vi "SIAM-SIMStack_v3.vi"(7 "Constants":T4={"galvox-Line0"=14895, "GalvoX-Blanking"=15500.0, "galvox-count/pix"=-2.474, "Camera-StartLine"=-62, "Camera-Endline"=4000, "Wobbel-total"=4264.0, "SM_ticks"=116, "Trigger_ticks"=100, "galvoxAccel"=5.0, "WobbelAccel"=0.02, "zAccel"=0.05, "z-delay-ticks"=700, "SCMOS-LineSpeed [10µs]"=2.4996, "RS height- Pix"=100, "extra-xgalvo"=83.0, "zcommand"=4026531840, "min turn ticks"=100.0} {"zcommand" format="%x" items=["end_no_ticket"=4027514895, "end_ticket"=4027518991, "NoOp"=4026531840, "Read ticks"=4026535936, "Read ticks to var"=4026535938, "Read IP"=4043313152, "Read IP into var"=4043313154, "Set IP from var"=4043309059, "Set IP from var, relative"=4043313155, "branchRel_if_equal"=4043374849, "decrement_branchRel_if_equal"=4043374945, "decrement_branchRel_if_greaterequal"=4043375201, "decrement_branchRel_if_greaterequal_withTicket"=4043379297, "decrement_branchRel_if_smaller"=4043375457, "increment_branchRel_if_smaller"=4043375473, "readVar"=4060090368, "writeVar"=4060086273, "copyVar0_from_var1"=4060086275, "math_addToVariable"=4076863488, "math_addVToVariable"=4076863489, "math_subToVariable"=4076863490, "math_subVToVariable"=4076863491, "math_multToVariable"=4076863492, "math_multvToVariable"=4076863493, "math_divideToVariable"=4076863494, "math_divideVToVariable"=4076863495, "math_modToVariable"=4076863496, "math_modVToVariable"=4076863497, "logic_and"=4093640704, "logic_or"=4093640706, "logic_xor"=4093640708, "bitshift"=4093640712, "I2C-write"=335544337, "I2C-read"=335548433, "Cam-SPI-write"=3254779905, "UART0-VC-Baud-write"=469958673, "UART0-VC-Baud-read"=469962768, "UART0-VC-write"=469762065, "UART0-VC-write-Var"=469762067, "UART0-VC-read-availabe-bytes-to-var"=470355970, "UART0-VC-read-availabe-bytes"=470355984, "UART0-VC-read-skip-bytes"=469831681, "UART0-VC-read"=469766160, "UART0-VC-read-Var"=469766162, "UART1-TSM-Baud-write"=486735889, "UART1-TSM-Baud-read"=486739984, "UART1-TSM-write"=486539281, "UART1-TSM-write-Var"=486539283, "UART1-TSM-read-availabe-bytes-to-var"=487133186, "UART1-TSM-read-availabe-bytes"=487133200, "UART1-TSM-read-skip-bytes"=486604801, "UART1-TSM-read-skip-bytes"=486608897, "UART1-TSM-read"=486543376, "UART1-TSM-read-Var"=486543378, "UART2-Laser-Baud-write"=503513105, "UART2-Baud-read"=503517200, "UART2-write"=503316497, "UART2-write-Var"=503316499, "UART2-read-availabe-bytes-to-var"=503910402, "UART2-read-availabe-bytes"=503910416, "UART2-read-skip-bytes"=503386113, "UART2-read"=503320592, "UART2-read-Var"=503320594, "UART3-Baud-write"=520290321, "UART3-Baud-read"=520294416, "UART3-write"=520093713, "UART3-write-Var"=520093715, "UART3-read-availabe-bytes-to-var"=520687618, "UART3-read-availabe-bytes"=520687632, "UART3-read-skip-bytes"=520163329, "UART3-read"=520097808, "UART3-read-Var"=520097810, "IO-read_bank0"=3489665024, "IO-write_bank0"=3489660929, "IO-read_bank1"=3506442240, "IO-write_bank1"=3506438145, "DA0-0_LED365"=2684354561, "DA0-1_LED385"=2685403137, "DA0-2_LED440"=2686451713, "DA0-3_LED470"=2687500289, "DA0-4_LED510"=2688548865, "DA0-5_LED550"=2689597441, "DA0-6_LED590"=2690646017, "DA0-7_LED640"=2691694593, "DA1-0_LED-R"=2701131777, "DA1-1_LED-G"=2702180353, "DA1-2_LED-B"=2703228929, "DA1-3_LED-AF"=2704277505, "DA1-4"=2705326081, "DA1-5"=2706374657, "DA1-6"=2707423233, "DA1-7"=2708471809, "DA2-Laser0"=2717908993, "DA2-Laser1"=2718957569, "DA2-Laser2"=2720006145, "DA2-Laser3"=2721054721, "DA2-Laser4"=2722103297, "Analog-read_AD0-0"=2818576384, "Analog-read-store_AD0-0"=2818572290, "AF-Register-transfer r/w"=2835349505, "AF-Register-read"=2835353600, "AF-Register-read-to-var"=2835353602, "AF-Transfer-from-var"=2835349507, "IO-delay_bank0"=3489923073, "IO-delay_bank0_fromVar"=3489923075, "read_cam_clock"=3289124864, "store_cam_clock"=3289120770, "read_cam_phase"=3289190400, "store_cam_phase"=3289186306, "store_cam_phase-t"=3289190402, "r_cam1_NHS"=3254980608, "w_cam1_NHS"=3254976513, "r_cam1_NVS"=3255046144, "w_cam1_NVS"=3255042049, "r_cam1_npx"=3255111680, "w_cam1_npx"=3255107585, "r_cam1_npy"=3255177216, "w_cam1_npy"=3255173121, "r_cam1_xhswait"=3255439360, "w_cam1_xhswait"=3255435265, "r_cam1_xvs_wait"=3255504896, "w_cam1_xvs_wait"=3255500801, "r_cam1_framcounter"=3255570432, "r_cam1_line"=3255635968, "r_cam1_xhs-counter"=3255701504, "r_cam2_NHS"=3271757824, "w_cam2_NHS"=3271753729, "r_cam2_NVS"=3271823360, "w_cam2_NVS"=3271819265, "r_cam2_npx"=3271888896, "w_cam2_npx"=3271884801, "r_cam2_npy"=3271954432, "w_cam2_npy"=3271950337, "r_cam2_xvs_wait"=3272282112, "w_cam2_xvs_wait"=3272278017, "r_cam2_framcounter"=3272347648, "r_cam2_line"=3272413184, "r_cam2_xhs-counter"=3272478720, "start TMSI"=102694919, "set_1Galvo"=101712113, "set_x-Galvo"=102760689, "set_y-Galvo"=103809265, "set_z-Fokus"=104857841, "set_1Galvo_position-only"=101711937, "set_x-Galvo_position-only"=102760513, "set_y-Galvo_position-only"=103809089, "set_z-Fokus_position-only"=104857665, "set_x-Galvo_position-only_ticket"=102764609, "set_y-Galvo_position-only_ticket"=103813185, "set_z-Fokus_position-only_ticket"=104861761, "set_1Galvo_relativ-only"=101712001, "set_x-Galvo_relativ-only"=102760577, "set_y-Galvo_relativ-only"=103809153, "set_z-Fokus_relativ-only"=104857729, "set_1Galvo_speed-only"=101711905, "set_x-Galvo_speed-only"=102760481, "set_y-Galvo_speed-only"=103809057, "set_z-Fokus_speed-only"=104857633, "set_1Galvo_acc-only"=101711889, "set_x-Galvo_acc-only"=102760465, "set_y-Galvo_acc-only"=103809041, "set_z-Fokus_acc-only"=104857617, "read_1Galvo_ticket"=101716032, "read_x-Galvo_ticket"=102764608, "read_y-Galvo_ticket"=103813184, "read_z-Focus_ticket"=104861760, "x-Galvo_pos_fromVar"=102760515, "y-Galvo_pos_fromVar"=103809091, "z-Focus_pos_fromVar"=104857667, "Servo0"=67108865, "Servo0-enable"=68091911, "Servo0-disable"=68091919, "Servo1"=68157441, "Servo1-enable"=69140487, "Servo1-disable"=69140495, "Servo2-enable"=70189063, "Servo2"=69206017, "Servo3-enable"=71237639, "Servo3"=70254593, "x-ssi-init"=202309639, "x-ssi-disable"=202309647, "x-ssi-Bits"=201523201, "x-ssi-Read"=201330688, "x-ssi-ReadToVar"=201326594, "x-ssi-ReadToVar-ticket"=201330690, "y-ssi-init"=203358215, "y-ssi-disable"=203358223, "y-ssi-Bits"=202571777, "y-ssi-Read"=202379264, "y-ssi-ReadToVar"=202375170, "y-ssi-ReadToVat-ticket"=202379266]; "SCMOS-LineSpeed [10µs]" format="%#.6f" items=["EdgeFast-285MHz"=0.9175, "EdgeSlow-95MHz"=2.7525, "Panda4.2"=2.7766, "mer2000"=2.4996]; "galvox-count/pix" format="%#_5f"}, 8 "error in (no error)":errorcluster, 11 "User":T5={"z-distance_motorunits"=100, "#planes"=1, "Digital-out"=enum."Laser1", "NoOfPhaseImages"=7} {"#planes" min=1}) -> (0 "error out":errorcluster, 1 "SIAMScript":T6(array[cluster])=[{"Delay 10µs"=50, "command"=4060086273, "P0"=3, "P1"=1, "P2"=0, "P3"=0, "P4"=0, "P5-ticket"=0, "comment"=""}, {"Delay 10µs"=0, "command"=101711937, "P0"=0, "P1"=160563200, "P2"=0, "P3"=0, "P4"=0, "P5-ticket"=0, "comment"=""}, {"Delay 10µs"=0, "command"=102760513, "P0"=0, "P1"=985958318, "P2"=0, "P3"=0, "P4"=0, "P5-ticket"=0, "comment"=""}, {"Delay 10µs"=0, "command"=3289190402, "P0"=0, "P1"=0, "P2"=0, "P3"=0, "P4"=0, "P5-ticket"=0, "comment"=""}, {"Delay 10µs"=1, "command"=4076863488, "P0"=0, "P1"=381040, "P2"=0, "P3"=0, "P4"=0, "P5-ticket"=0, "comment"=""}, {"Delay 10µs"=0, "command"=4076863492, "P0"=0, "P1"=0, "P2"=0, "P3"=0, "P4"=0, "P5-ticket"=0, "comment"=""}, {"Delay 10µs"=0, "command"=4076863497, "P0"=0, "P1"=1, "P2"=0, "P3"=0, "P4"=0, "P5-ticket"=0, "comment"=""}, {"Delay 10µs"=0, "command"=4076863494, "P0"=0, "P1"=0, "P2"=0, "P3"=0, "P4"=0, "P5-ticket"=0, "comment"=""}, {"Delay 10µs"=0, "command"=4076863488, "P0"=0, "P1"=40, "P2"=0, "P3"=0, "P4"=0, "P5-ticket"=0, "comment"=""}, {"Delay 10µs"=0, "command"=4060086273, "P0"=10, "P1"=-65, "P2"=0, "P3"=0, "P4"=0, "P5-ticket"=0, "comment"=""}, {"Delay 10µs"=0, "command"=4076863492, "P0"=10, "P1"=0, "P2"=0, "P3"=0, "P4"=0, "P5-ticket"=0, "comment"=""}, {"Delay 10µs"=264, "command"=102760481, "P0"=0, "P1"=0, "P2"=-1047728, "P3"=0, "P4"=0, "P5-ticket"=0, "comment"=""}, {"Delay 10µs"=0, "command"=4060086273, "P0"=2, "P1"=7, "P2"=0, "P3"=0, "P4"=0, "P5-ticket"=0, "comment"=""}, {"Delay 10µs"=116, "command"=3489660929, "P0"=2097152, "P1"=2097152, "P2"=0, "P3"=0, "P4"=0, "P5-ticket"=0, "comment"=""}, {"Delay 10µs"=0, "command"=3489660929, "P0"=1, "P1"=1, "P2"=0, "P3"=0, "P4"=0, "P5-ticket"=0, "comment"=""}, {"Delay 10µs"=100, "command"=3489660929, "P0"=1, "P1"=0, "P2"=0, "P3"=0, "P4"=0, "P5-ticket"=0, "comment"=""}, {"Delay 10µs"=12638, "command"=3289190402, "P0"=0, "P1"=0, "P2"=0, "P3"=0, "P4"=0, "P5-ticket"=0, "comment"=""}, {"Delay 10µs"=1, "command"=4076863488, "P0"=0, "P1"=381040, "P2"=0, "P3"=0, "P4"=0, "P5-ticket"=0, "comment"=""}, {"Delay 10µs"=0, "command"=4076863492, "P0"=0, "P1"=0, "P2"=0, "P3"=0, "P4"=0, "P5-ticket"=0, "comment"=""}, {"Delay 10µs"=0, "command"=4076863497, "P0"=0, "P1"=1, "P2"=0, "P3"=0, "P4"=0, "P5-ticket"=0, "comment"=""}, {"Delay 10µs"=0, "command"=4076863494, "P0"=0, "P1"=0, "P2"=0, "P3"=0, "P4"=0, "P5-ticket"=0, "comment"=""}, {"Delay 10µs"=0, "command"=4076863488, "P0"=0, "P1"=40, "P2"=0, "P3"=0, "P4"=0, "P5-ticket"=0, "comment"=""}, {"Delay 10µs"=0, "command"=4060086273, "P0"=10, "P1"=-65, "P2"=0, "P3"=0, "P4"=0, "P5-ticket"=0, "comment"=""}, {"Delay 10µs"=0, "command"=4076863492, "P0"=10, "P1"=0, "P2"=0, "P3"=0, "P4"=0, "P5-ticket"=0, "comment"=""}, {"Delay 10µs"=0, "command"=102760465, "P0"=0, "P1"=794884, "P2"=0, "P3"=0, "P4"=0, "P5-ticket"=0, "comment"=""}, {"Delay 10µs"=0, "command"=101711889, "P0"=0, "P1"=42448, "P2"=0, "P3"=0, "P4"=0, "P5-ticket"=0, "comment"=""}, {"Delay 10µs"=132, "command"=102760465, "P0"=0, "P1"=-794884, "P2"=0, "P3"=0, "P4"=0, "P5-ticket"=0, "comment"=""}, {"Delay 10µs"=0, "command"=101711889, "P0"=0, "P1"=-42448, "P2"=0, "P3"=0, "P4"=0, "P5-ticket"=0, "comment"=""}, {"Delay 10µs"=132, "command"=102760465, "P0"=0, "P1"=0, "P2"=0, "P3"=0, "P4"=0, "P5-ticket"=0, "comment"=""}, {"Delay 10µs"=0, "command"=101711889, "P0"=0, "P1"=0, "P2"=0, "P3"=0, "P4"=0, "P5-ticket"=0, "comment"=""}, {"Delay 10µs"=12855, "command"=3489660929, "P0"=2097152, "P1"=0, "P2"=0, "P3"=0, "P4"=0, "P5-ticket"=0, "comment"=""}, {"Delay 10µs"=70, "command"=4043379297, "P0"=-6, "P1"=2, "P2"=1, "P3"=0, "P4"=0, "P5-ticket"=514, "comment"=""}, {"Delay 10µs"=50, "command"=104857729, "P0"=-25600, "P1"=0, "P2"=0, "P3"=0, "P4"=0, "P5-ticket"=0, "comment"=""}, {"Delay 10µs"=0, "command"=4043379297, "P0"=-43, "P1"=3, "P2"=1, "P3"=0, "P4"=0, "P5-ticket"=515, "comment"=""}, {"Delay 10µs"=50, "command"=104857729, "P0"=25600, "P1"=0, "P2"=0, "P3"=0, "P4"=0, "P5-ticket"=0, "comment"=""}, {"Delay 10µs"=50, "command"=102760513, "P0"=0, "P1"=983040000, "P2"=0, "P3"=0, "P4"=0, "P5-ticket"=0, "comment"=""}, {"Delay 10µs"=10, "command"=4027518991, "P0"=0, "P1"=0, "P2"=0, "P3"=0, "P4"=0, "P5-ticket"=112, "comment"=""}] {"command" format="%x" items=["end_no_ticket"=4027514895, "end_ticket"=4027518991, "NoOp"=4026531840, "Read ticks"=4026535936, "Read ticks to var"=4026535938, "Read IP"=4043313152, "Read IP into var"=4043313154, "Set IP from var"=4043309059, "Set IP from var, relative"=4043313155, "branchRel_if_equal"=4043374849, "decrement_branchRel_if_equal"=4043374945, "decrement_branchRel_if_greaterequal"=4043375201, "decrement_branchRel_if_greaterequal_withTicket"=4043379297, "decrement_branchRel_if_smaller"=4043375457, "increment_branchRel_if_smaller"=4043375473, "readVar"=4060090368, "writeVar"=4060086273, "copyVar0_from_var1"=4060086275, "math_addToVariable"=4076863488, "math_addVToVariable"=4076863489, "math_subToVariable"=4076863490, "math_subVToVariable"=4076863491, "math_multToVariable"=4076863492, "math_multvToVariable"=4076863493, "math_divideToVariable"=4076863494, "math_divideVToVariable"=4076863495, "math_modToVariable"=4076863496, "math_modVToVariable"=4076863497, "logic_and"=4093640704, "logic_or"=4093640706, "logic_xor"=4093640708, "bitshift"=4093640712, "I2C-write"=335544337, "I2C-read"=335548433, "Cam-SPI-write"=3254779905, "UART0-VC-Baud-write"=469958673, "UART0-VC-Baud-read"=469962768, "UART0-VC-write"=469762065, "UART0-VC-write-Var"=469762067, "UART0-VC-read-availabe-bytes-to-var"=470355970, "UART0-VC-read-availabe-bytes"=470355984, "UART0-VC-read-skip-bytes"=469831681, "UART0-VC-read"=469766160, "UART0-VC-read-Var"=469766162, "UART1-TSM-Baud-write"=486735889, "UART1-TSM-Baud-read"=486739984, "UART1-TSM-write"=486539281, "UART1-TSM-write-Var"=486539283, "UART1-TSM-read-availabe-bytes-to-var"=487133186, "UART1-TSM-read-availabe-bytes"=487133200, "UART1-TSM-read-skip-bytes"=486604801, "UART1-TSM-read-skip-bytes"=486608897, "UART1-TSM-read"=486543376, "UART1-TSM-read-Var"=486543378, "UART2-Laser-Baud-write"=503513105, "UART2-Baud-read"=503517200, "UART2-write"=503316497, "UART2-write-Var"=503316499, "UART2-read-availabe-bytes-to-var"=503910402, "UART2-read-availabe-bytes"=503910416, "UART2-read-skip-bytes"=503386113, "UART2-read"=503320592, "UART2-read-Var"=503320594, "UART3-Baud-write"=520290321, "UART3-Baud-read"=520294416, "UART3-write"=520093713, "UART3-write-Var"=520093715, "UART3-read-availabe-bytes-to-var"=520687618, "UART3-read-availabe-bytes"=520687632, "UART3-read-skip-bytes"=520163329, "UART3-read"=520097808, "UART3-read-Var"=520097810, "IO-read_bank0"=3489665024, "IO-write_bank0"=3489660929, "IO-read_bank1"=3506442240, "IO-write_bank1"=3506438145, "DA0-0_LED365"=2684354561, "DA0-1_LED385"=2685403137, "DA0-2_LED440"=2686451713, "DA0-3_LED470"=2687500289, "DA0-4_LED510"=2688548865, "DA0-5_LED550"=2689597441, "DA0-6_LED590"=2690646017, "DA0-7_LED640"=2691694593, "DA1-0_LED-R"=2701131777, "DA1-1_LED-G"=2702180353, "DA1-2_LED-B"=2703228929, "DA1-3_LED-AF"=2704277505, "DA1-4"=2705326081, "DA1-5"=2706374657, "DA1-6"=2707423233, "DA1-7"=2708471809, "DA2-Laser0"=2717908993, "DA2-Laser1"=2718957569, "DA2-Laser2"=2720006145, "DA2-Laser3"=2721054721, "DA2-Laser4"=2722103297, "Analog-read_AD0-0"=2818576384, "Analog-read-store_AD0-0"=2818572290, "AF-Register-transfer r/w"=2835349505, "AF-Register-read"=2835353600, "AF-Register-read-to-var"=2835353602, "AF-Transfer-from-var"=2835349507, "IO-delay_bank0"=3489923073, "IO-delay_bank0_fromVar"=3489923075, "read_cam_clock"=3289124864, "store_cam_clock"=3289120770, "read_cam_phase"=3289190400, "store_cam_phase"=3289186306, "store_cam_phase-t"=3289190402, "r_cam1_NHS"=3254980608, "w_cam1_NHS"=3254976513, "r_cam1_NVS"=3255046144, "w_cam1_NVS"=3255042049, "r_cam1_npx"=3255111680, "w_cam1_npx"=3255107585, "r_cam1_npy"=3255177216, "w_cam1_npy"=3255173121, "r_cam1_xhswait"=3255439360, "w_cam1_xhswait"=3255435265, "r_cam1_xvs_wait"=3255504896, "w_cam1_xvs_wait"=3255500801, "r_cam1_framcounter"=3255570432, "r_cam1_line"=3255635968, "r_cam1_xhs-counter"=3255701504, "r_cam2_NHS"=3271757824, "w_cam2_NHS"=3271753729, "r_cam2_NVS"=3271823360, "w_cam2_NVS"=3271819265, "r_cam2_npx"=3271888896, "w_cam2_npx"=3271884801, "r_cam2_npy"=3271954432, "w_cam2_npy"=3271950337, "r_cam2_xvs_wait"=3272282112, "w_cam2_xvs_wait"=3272278017, "r_cam2_framcounter"=3272347648, "r_cam2_line"=3272413184, "r_cam2_xhs-counter"=3272478720, "start TMSI"=102694919, "set_1Galvo"=101712113, "set_x-Galvo"=102760689, "set_y-Galvo"=103809265, "set_z-Fokus"=104857841, "set_1Galvo_position-only"=101711937, "set_x-Galvo_position-only"=102760513, "set_y-Galvo_position-only"=103809089, "set_z-Fokus_position-only"=104857665, "set_x-Galvo_position-only_ticket"=102764609, "set_y-Galvo_position-only_ticket"=103813185, "set_z-Fokus_position-only_ticket"=104861761, "set_1Galvo_relativ-only"=101712001, "set_x-Galvo_relativ-only"=102760577, "set_y-Galvo_relativ-only"=103809153, "set_z-Fokus_relativ-only"=104857729, "set_1Galvo_speed-only"=101711905, "set_x-Galvo_speed-only"=102760481, "set_y-Galvo_speed-only"=103809057, "set_z-Fokus_speed-only"=104857633, "set_1Galvo_acc-only"=101711889, "set_x-Galvo_acc-only"=102760465, "set_y-Galvo_acc-only"=103809041, "set_z-Fokus_acc-only"=104857617, "read_1Galvo_ticket"=101716032, "read_x-Galvo_ticket"=102764608, "read_y-Galvo_ticket"=103813184, "read_z-Focus_ticket"=104861760, "x-Galvo_pos_fromVar"=102760515, "y-Galvo_pos_fromVar"=103809091, "z-Focus_pos_fromVar"=104857667, "Servo0"=67108865, "Servo0-enable"=68091911, "Servo0-disable"=68091919, "Servo1"=68157441, "Servo1-enable"=69140487, "Servo1-disable"=69140495, "Servo2-enable"=70189063, "Servo2"=69206017, "Servo3-enable"=71237639, "Servo3"=70254593, "x-ssi-init"=202309639, "x-ssi-disable"=202309647, "x-ssi-Bits"=201523201, "x-ssi-Read"=201330688, "x-ssi-ReadToVar"=201326594, "x-ssi-ReadToVar-ticket"=201330690, "y-ssi-init"=203358215, "y-ssi-disable"=203358223, "y-ssi-Bits"=202571777, "y-ssi-Read"=202379264, "y-ssi-ReadToVar"=202375170, "y-ssi-ReadToVat-ticket"=202379266]}, 2 "Camera":T2={"Camera-Expos ms"=0.0, "CameraImages"=7, "cam fps min."=0.0})   [LabVIEW 2011]
uses:
  SIAM_command.ctl
panel:
  in  "calulate values for debug":bool
  out "Waveform Graph":dbl[][](graph)
  in  "Aktiv":T1(array[ring])=[enum."GalvoX", enum."Galvo4"]
  out "phase a":dbl=0.04048114735137636
  out "galvo a":dbl=0.7580607172293603
  out "xGalvoMove":dbl=-12844.599514563108
  out "FrameClock":u32=13119
  out "CamTics":u32=12855
  out "x vel":dbl=-0.9991909385113269
  out "~x-move":dbl=12841.530000000002
  out "~xgalvoend":dbl=2202.999999999998
  out "xgalvostart":dbl=15044.53
  out "expected xduration":dbl=71.67016115511393
  out "expected  Wduration":dbl=264.5751311064591
  out "size(s)":i32=37
  out "WobSubShift":dbl=700.0
  out "Half Turn_ticks":u32=132
  # "version ohne phase!\nversion mit galvo1 parallel galvox!: extra-xgalvo\ntodo: exact interger calculation\ntodo: remove last wobber shift from loop\nlost images? increas min turn ticks\nslow z: increse z-delay"
  # "var 2 =linecounter \nvar 3 =framecounter"
  # "tmsi motor units is *512nm, flumias2020 *~5nm"
  # "<-- user inputs --------------------------- constants ---->"
  # "debug disabled if good working"
  # "15173"
  # "naja nicht immer konstante\nalles count und Pixel und 10µs !!!"
  # "wobbler shift(7)=SQRT(7)*pitch"
  # "lineclock read slow=AD99E =711070 =/256=27.77617"
  # "a gerechnet wobbler~3.7, x~98, eher /10\nz~6ms/2µm"
  # "shift full phase"
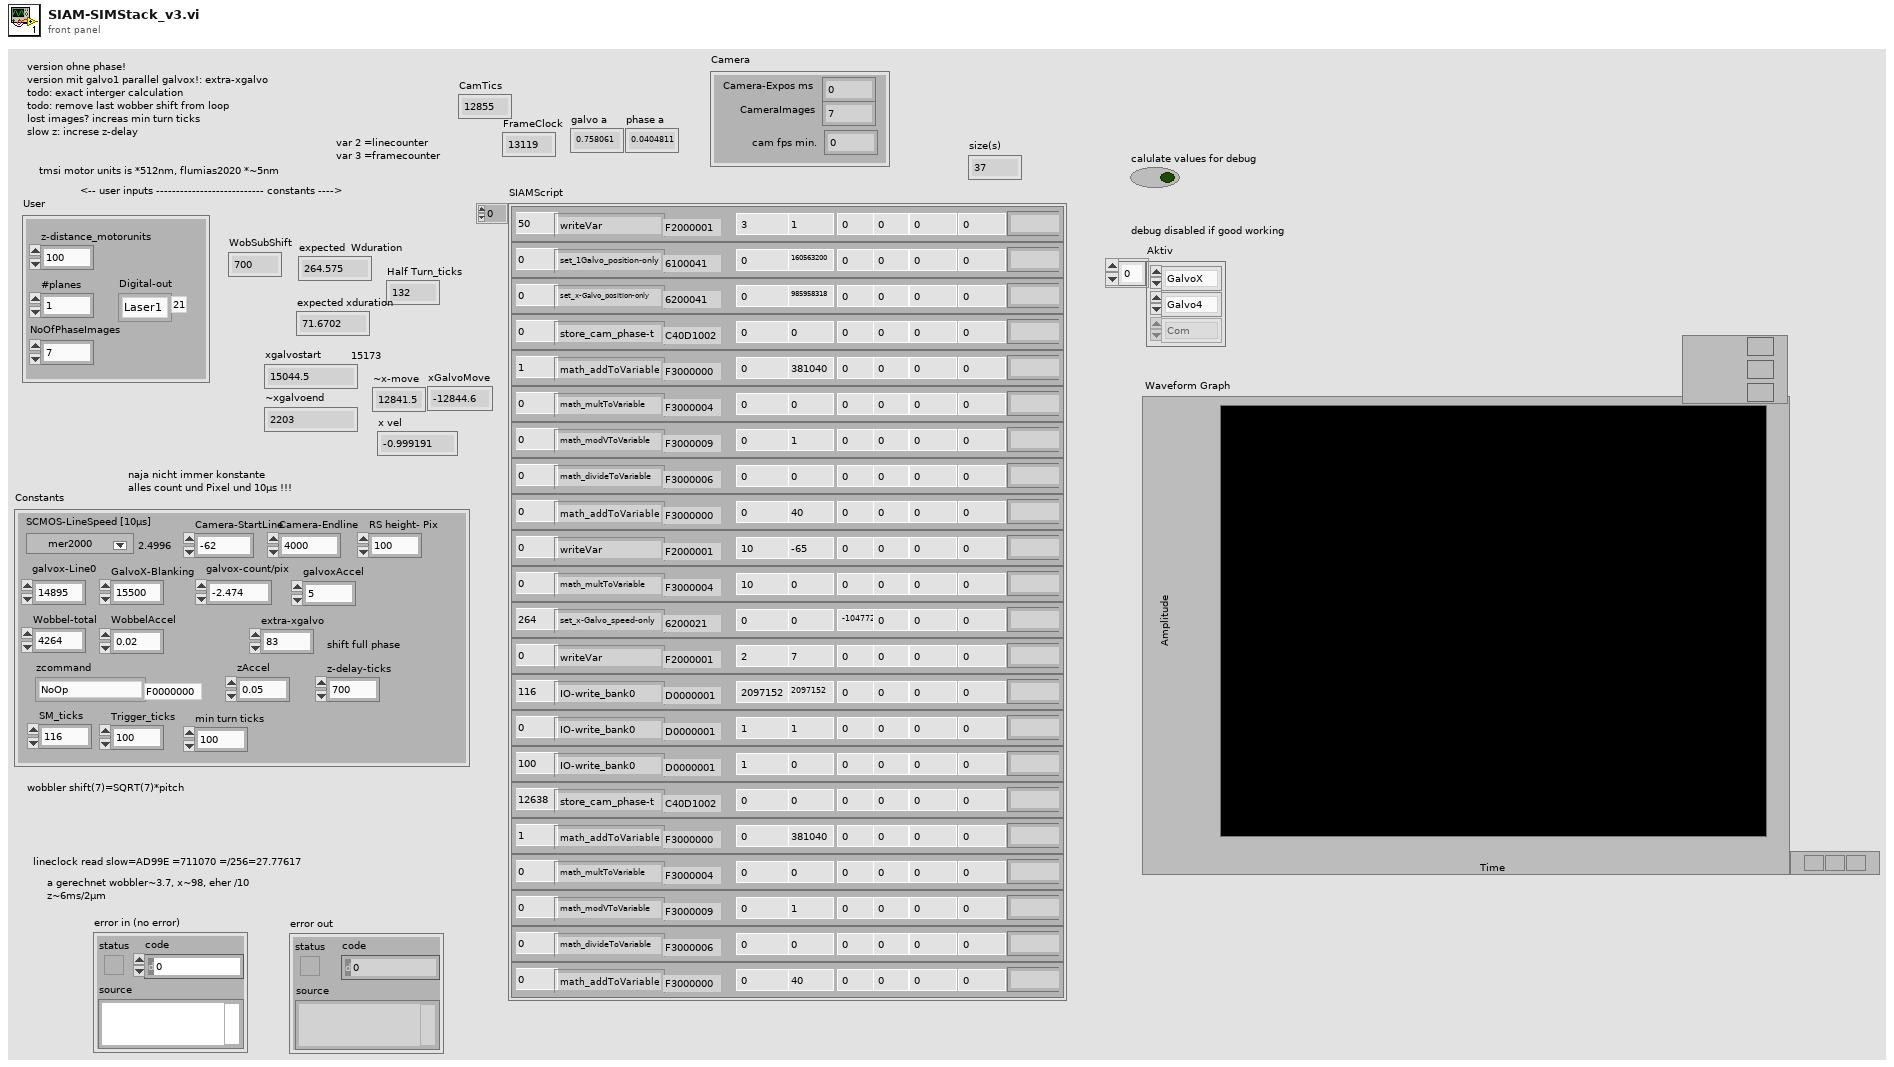
[diagram p1: front panel]
types:
  T1 = enum16{"Com", "AnalogConfig", "AnalogValue", "GalvoX", "GalvoY", "Galvo3", "Galvo4", "Digital", "Free", "Loop", "SMoveTime", "Image1X", "Image1Y", "Image2X", "Image2Y"}[]
  T2 = cluster{"Camera-Expos ms":dbl, "CameraImages":u16, "cam fps min.":dbl}
  T3 = typedef "SIAM_command.ctl" = u32
  T4 = cluster{"galvox-Line0":i16, "GalvoX-Blanking":dbl, "galvox-count/pix":dbl, "Camera-StartLine":i32, "Camera-Endline":u32, "Wobbel-total":dbl, "SM_ticks":u32, "Trigger_ticks":u32, "galvoxAccel":dbl, "WobbelAccel":dbl, "zAccel":dbl, "z-delay-ticks":u32, "SCMOS-LineSpeed [10µs]":dbl, "RS height- Pix":u16, "extra-xgalvo":dbl, "zcommand":T3, "min turn ticks":dbl}
  T5 = cluster{"z-distance_motorunits":i32, "#planes":u16, "Digital-out":enum8{"cam1", "cam1-ready?", "cam2", "cam2-ready?", "tmsx?", "tsmy?", "tsm3?", "lid?", "led1", "led2", "led3", "led4", "led5", "led6", "led7", "led8", "durchR", "durchG", "durchB", "AF", "Laser0", "Laser1", "Laser2", "Laser3", "Laser4", "LaserX", "TrigOut", "SMB1", ""}, "NoOfPhaseImages":u16}
  T6 = cluster{"Delay 10µs":u32, "command":T3, "P0":i32, "P1":i32, "P2":i32, "P3":i32, "P4":i32, "P5-ticket":i32, "comment":string}[]
  T7 = enum8{"Ch0", "Ch1", "x-Galvo", "y-Galvo", "z-Focus"}
  T8 = cluster{"Delay 10µs":u32, "command":T3, "P0":i32, "P1":i32, "P2":i32, "P3":i32, "P4":i32, "P5-ticket":i32, "comment":string}
  T9 = cluster{"Delay 10µs":u32, "command":T3, "P0":i32, "P1":i32, "P2":i32, "P3":i32, "P4":i32, "P5-ticket":i32}[]
  T10 = enum8{"cam1", "cam1-ready?", "cam2", "cam2-ready?", "tmsx?", "tsmy?", "tsm3?", "lid?", "led1", "led2", "led3", "led4", "led5", "led6", "led7", "led8", "durchR", "durchG", "durchB", "AF", "Laser0", "Laser1", "Laser2", "Laser3", "Laser4", "LaserX", "TrigOut", "SMB1", ""}
  T11 = cluster{"Delay 10µs":u32, "command":T3, "P0":i32, "P1":i32, "P2":i32, "P3":i32, "P4":i32, "P5-ticket":i32}
  T12 = typedef "ScanControl_Action.ctl" = enum16{"Abs", "Rel", "Inc", "IncInc", "LoopStart", "LoopEnd", "WaitTriggerRising"}
  T13 = typedef "ScanControl_Channel.ctl" = enum16{"Com", "AnalogConfig", "AnalogValue", "GalvoX", "GalvoY", "Galvo3", "Galvo4", "Digital", "Free", "Loop", "SMoveTime", "Image1X", "Image1Y", "Image2X", "Image2Y"}
  T14 = cluster{"Time [10µs]":dbl, "action":T12, "channel":T13, "value (/s)":dbl}[]
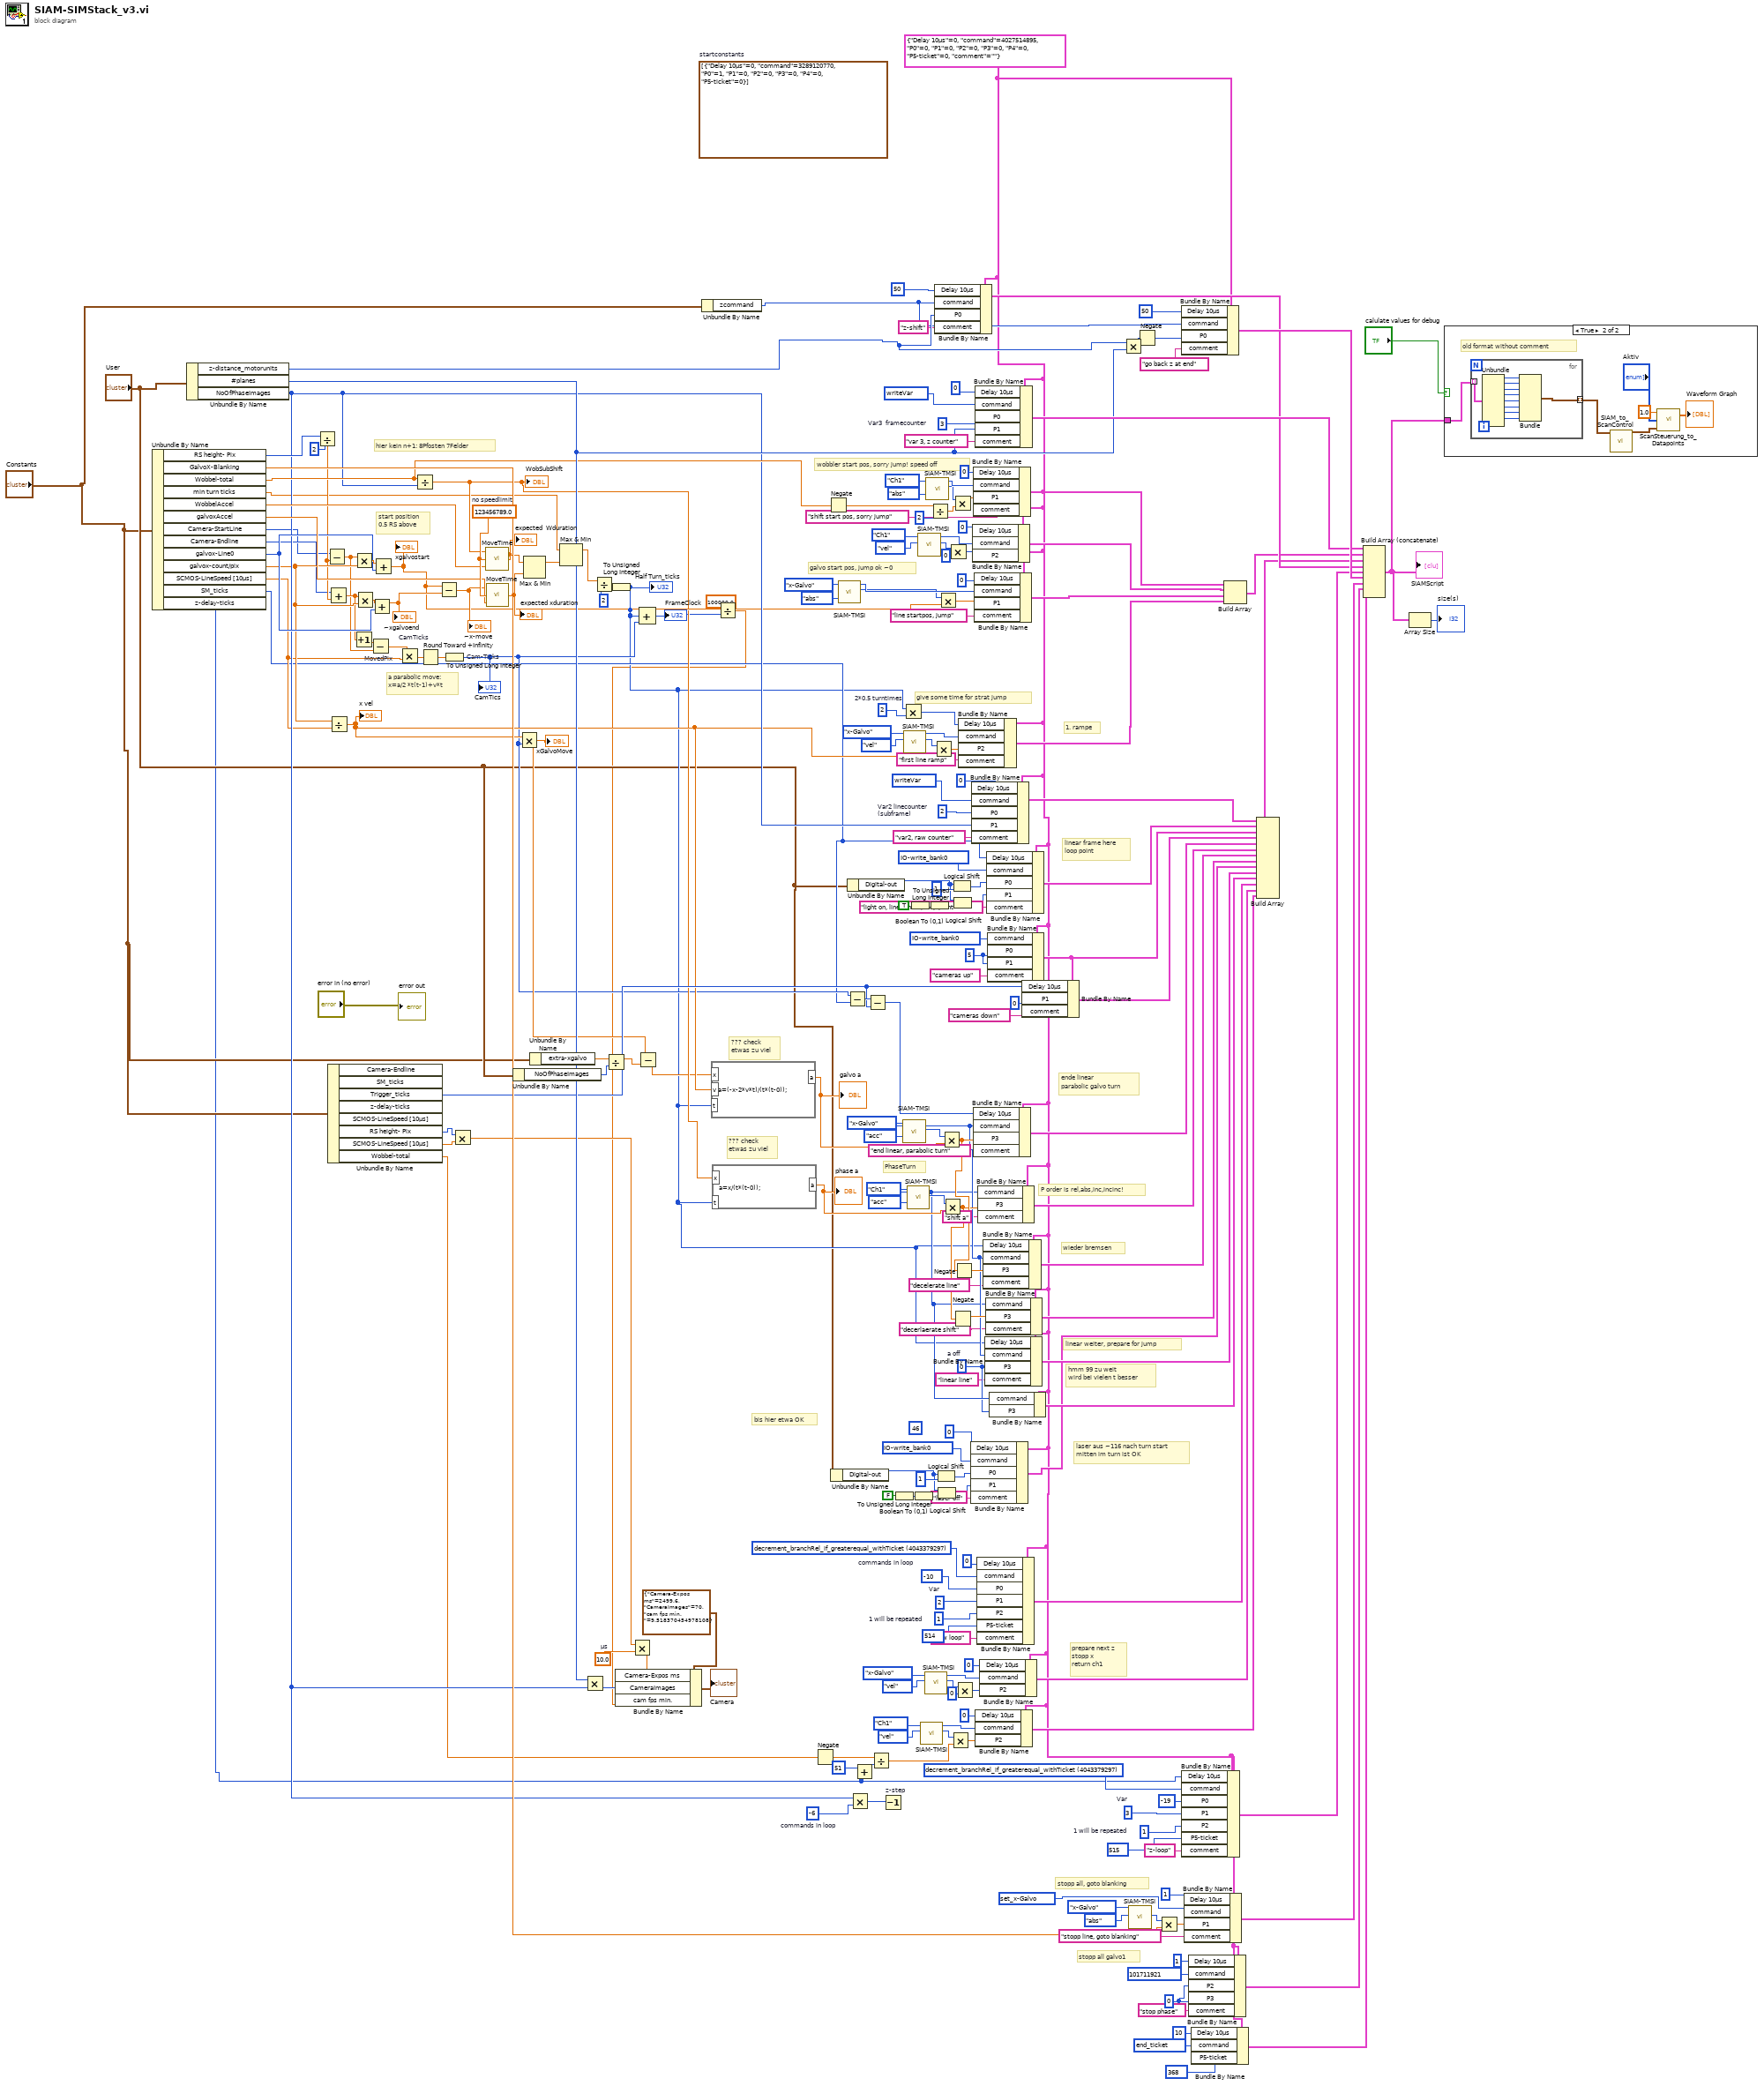
[diagram p0: block diagram]
diagram:
  w24 = 0 ("P2")
  w27 = T3 101711921 items=["read_x-Motor_status_ticket"=17305600, "init_x-Motor"=17760263, "read_x-Motor_absolute_ticket"=16781312, "move_x-Motor_absolute"=16777217, "move_x-Motor_relative"=16842753, "read_x-Motor_speed"=16977920, "set_x-Motor_speed"=16973825, "read_y-Motor_status_ticket"=18354176, "init_y-Motor"=18808839, "read_y-Motor_absolute_ticket"=17829888, "move_y-Motor_absolute"=17825793, "move_y-Motor_relative"=17891329, "read_y-Motor_speed"=18026496, "set_y-Motor_speed"=18022401, "read_z-Motor_status_ticket"=19402752, "init_z-Motor"=19857415, "stop_z-Motor"=19857423, "start_z-Motor"=19857422, "read_z-Motor_absolute_ticket"=18878464, "move_z-Motor_absolute"=18874369, "move_z-Motor_relative"=18939905, "read_Objective_status_ticket"=20451328, "init_Objective"=20905991, "read_Objective_absolute_ticket"=19927040, "move_Objective_absolute"=19922945, "move_Objective_relative"=19988481, "read_Objective-Motor_speed"=20123648, "set_Objective-Motor_speed"=20119553, "read_Filter_status_ticket"=21499904, "init_Filter"=21954567, "read_Filter_absolute_ticket"=20975616, "move_Filter_absolute"=20971521, "move_Filter_relative"=21037057, "read_Filter-Motor_speed"=21172224, "set_Filter-Motor_speed"=21168129, "read_Trans-Rad_status_ticket"=22548480, "init_Trans-Rad"=23003143, "read_Trans-Rad_absolute_ticket"=22024192, "move_Trans-Rad_absolute"=22020097, "move_Trans-Rad_relative"=22085633, "read_Trans-Motor_speed"=22220800, "set_Trans-Motor_speed"=22216705, "read_FRET_status_ticket"=23597056, "init_FRET"=24051719, "read_FRET_absolute_ticket"=23072768, "move_FRET_absolute"=23068673, "move_FRET_relative"=23134209, "read_FRET-Motor_speed"=23269376, "set_FRET-Motor_speed"=23265281, "read_SI-Rad_status_ticket"=24645632, "init_SI-Rad"=25100295, "read_SI-Rad_absolute_ticket"=24121344, "move_SI-Rad_absolute"=24117249, "move_SI-Rad_relative"=24182785, "read_SI-Rad_speed"=24317952, "set_SI-Rad_speed"=24313857, "I2C-write"=335544337, "I2C-read"=335548433, "UART0-VC-Baud-write"=469958673, "UART0-VC-Baud-read"=469962768, "UART0-VC-write"=469762065, "UART0-VC-write-Var"=469762067, "UART0-VC-read"=469766160, "UART0-VC-read-Var"=469766162, "UART1-TSM-Baud-read"=486739984, "UART1-TSM-write"=486539281, "UART1-TSM-write-ticket"=486543377, "UART1-TSM-write-var-binary"=486539283, "UART1-TSM-write-var-binary-ticket"=486543379, "UART1-TSM-read"=486543376, "UART1-TSM-read-var-binary"=486543378, "UART2-write"=503316497, "UART2-read"=503320592, "USB-UART0-write"=536870929, "USB-UART0-read"=536875024, "USB-UART0-Float-Bitschift"=537133073, "USB-UART0-read-Float"=536875234, "USB-UART0-write-Float"=536871139, "USB-UART0-read-Float"=536875250, "USB-UART0-write-Float"=536871155, "end_no_ticket"=4027514895, "end_ticket"=4027518991, "NoOp"=4060086272, "IO-read_bank0"=3489665024, "IO-write_bank0"=3489660929, "IO-read_bank1"=3506442240, "IO-write_bank1"=3506438145, "DA0-0_LED365"=2684354561, "DA0-1_LED385"=2685403137, "DA0-2_LED440"=2686451713, "DA0-3_LED470"=2687500289, "DA0-4_LED510"=2688548865, "DA0-5_LED550"=2689597441, "DA0-6_LED590"=2690646017, "DA0-7_LED640"=2691694593, "DA1-0_LED-R"=2701131777, "DA1-1_LED-G"=2702180353, "DA1-2_LED-B"=2703228929, "DA1-3_LED-AF"=2704277505, "DA1-4"=2705326081, "DA1-5"=2706374657, "DA1-6"=2707423233, "DA1-7"=2708471809, "DA2-Laser0"=2717908993, "DA2-Laser1"=2718957569, "DA2-Laser2"=2720006145, "DA2-Laser3"=2721054721, "DA2-Laser4"=2722103297, "Analog-read_AD0-0"=2818576384, "Analog-read-store_AD0-0"=2818572290, "IO-delay_bank0"=3489923073, "IO-delay_bank0_fromVar"=3489923075, "read_cam_clock"=3289124864, "store_cam_clock"=3289120770, "read_cam_phase"=3289190400, "store_cam_phase"=3289186306, "store_cam_phase-t"=3289190402, "Read ticks"=4026535936, "Read ticks to var"=4026535938, "Read IP"=4043313152, "Read IP into var"=4043313154, "Set IP from var"=4043309059, "Set IP from var, relative"=4043313155, "branchRel_if_equal"=4043374849, "decrement_branchRel_if_equal"=4043374945, "decrement_branchRel_if_greaterequal"=4043375201, "decrement_branchRel_if_greaterequal_withTicket"=4043379297, "decrement_branchRel_if_smaller"=4043375457, "increment_branchRel_if_smaller"=4043375473, "readVar"=4060090368, "writeVar"=4060086273, "copyVar0_from_var1"=4060086275, "math_addToVariable"=4076863488, "math_addVToVariable"=4076863489, "math_subToVariable"=4076863490, "math_subVToVariable"=4076863491, "math_multToVariable"=4076863492, "math_multvToVariable"=4076863493, "math_divideToVariable"=4076863494, "math_divideVToVariable"=4076863495, "math_modToVariable"=4076863496, "math_modVToVariable"=4076863497, "logic_and"=4093640704, "logic_or"=4093640706, "logic_xor"=4093640708, "bitshift"=4093640712, "set_1Galvo"=101712113, "set_x-Galvo"=102760689, "set_y-Galvo"=103809265, "set_z-Fokus"=104857841, "set_1Galvo_position-only"=101711937, "set_x-Galvo_position-only"=102760513, "set_y-Galvo_position-only"=103809089, "set_z-Fokus_position-only"=104857665, "set_x-Galvo_position-only_ticket"=102764609, "set_y-Galvo_position-only_ticket"=103813185, "set_z-Fokus_position-only_ticket"=104861761, "set_1Galvo_relativ-only"=101712001, "set_x-Galvo_relativ-only"=102760577, "set_y-Galvo_relativ-only"=103809153, "set_z-Fokus_relativ-only"=104857729, "set_1Galvo_speed-only"=101711905, "set_x-Galvo_speed-only"=102760481, "set_y-Galvo_speed-only"=103809057, "set_z-Fokus_speed-only"=104857633, "set_1Galvo_acc-only"=101711889, "set_x-Galvo_acc-only"=102760465, "set_y-Galvo_acc-only"=103809041, "set_z-Fokus_acc-only"=104857617, "read_1Galvo_ticket"=101716032, "read_x-Galvo_ticket"=102764608, "read_y-Galvo_ticket"=103813184, "read_z-Focus_ticket"=104861760, "x-Galvo_pos_fromVar"=102760515, "y-Galvo_pos_fromVar"=103809091, "z-Focus_pos_fromVar"=104857667, "Servo0"=67108865, "Servo0-enable"=68091911, "Servo0-disable"=68091919, "Servo1"=68157441, "Servo1-enable"=69140487, "Servo1-disable"=69140495, "Servo2-enable"=70189063, "Servo2"=69206017, "Servo3-enable"=71237639, "Servo3"=70254593, "x-ssi-init"=202309639, "x-ssi-disable"=202309647, "x-ssi-Bits"=201523201, "x-ssi-Read"=201330688, "x-ssi-ReadToVar"=201326594, "x-ssi-ReadToVar-ticket"=201330690, "y-ssi-init"=203358215, "y-ssi-disable"=203358223, "y-ssi-Bits"=202571777, "y-ssi-Read"=202379264, "y-ssi-ReadToVar"=202375170, "y-ssi-ReadToVat-ticket"=202379266] ("command")
  w29 = T3 102760689 items=["read_x-Motor_status_ticket"=17305600, "init_x-Motor"=17760263, "read_x-Motor_absolute_ticket"=16781312, "move_x-Motor_absolute"=16777217, "move_x-Motor_relative"=16842753, "read_x-Motor_speed"=16977920, "set_x-Motor_speed"=16973825, "read_y-Motor_status_ticket"=18354176, "init_y-Motor"=18808839, "read_y-Motor_absolute_ticket"=17829888, "move_y-Motor_absolute"=17825793, "move_y-Motor_relative"=17891329, "read_y-Motor_speed"=18026496, "set_y-Motor_speed"=18022401, "read_z-Motor_status_ticket"=19402752, "init_z-Motor"=19857415, "stop_z-Motor"=19857423, "start_z-Motor"=19857422, "read_z-Motor_absolute_ticket"=18878464, "move_z-Motor_absolute"=18874369, "move_z-Motor_relative"=18939905, "read_Objective_status_ticket"=20451328, "init_Objective"=20905991, "read_Objective_absolute_ticket"=19927040, "move_Objective_absolute"=19922945, "move_Objective_relative"=19988481, "read_Objective-Motor_speed"=20123648, "set_Objective-Motor_speed"=20119553, "read_Filter_status_ticket"=21499904, "init_Filter"=21954567, "read_Filter_absolute_ticket"=20975616, "move_Filter_absolute"=20971521, "move_Filter_relative"=21037057, "read_Filter-Motor_speed"=21172224, "set_Filter-Motor_speed"=21168129, "read_Trans-Rad_status_ticket"=22548480, "init_Trans-Rad"=23003143, "read_Trans-Rad_absolute_ticket"=22024192, "move_Trans-Rad_absolute"=22020097, "move_Trans-Rad_relative"=22085633, "read_Trans-Motor_speed"=22220800, "set_Trans-Motor_speed"=22216705, "read_FRET_status_ticket"=23597056, "init_FRET"=24051719, "read_FRET_absolute_ticket"=23072768, "move_FRET_absolute"=23068673, "move_FRET_relative"=23134209, "read_FRET-Motor_speed"=23269376, "set_FRET-Motor_speed"=23265281, "read_SI-Rad_status_ticket"=24645632, "init_SI-Rad"=25100295, "read_SI-Rad_absolute_ticket"=24121344, "move_SI-Rad_absolute"=24117249, "move_SI-Rad_relative"=24182785, "read_SI-Rad_speed"=24317952, "set_SI-Rad_speed"=24313857, "I2C-write"=335544337, "I2C-read"=335548433, "UART0-VC-Baud-write"=469958673, "UART0-VC-Baud-read"=469962768, "UART0-VC-write"=469762065, "UART0-VC-write-Var"=469762067, "UART0-VC-read"=469766160, "UART0-VC-read-Var"=469766162, "UART1-TSM-Baud-read"=486739984, "UART1-TSM-write"=486539281, "UART1-TSM-write-ticket"=486543377, "UART1-TSM-write-var-binary"=486539283, "UART1-TSM-write-var-binary-ticket"=486543379, "UART1-TSM-read"=486543376, "UART1-TSM-read-var-binary"=486543378, "UART2-write"=503316497, "UART2-read"=503320592, "USB-UART0-write"=536870929, "USB-UART0-read"=536875024, "USB-UART0-Float-Bitschift"=537133073, "USB-UART0-read-Float"=536875234, "USB-UART0-write-Float"=536871139, "USB-UART0-read-Float"=536875250, "USB-UART0-write-Float"=536871155, "end_no_ticket"=4027514895, "end_ticket"=4027518991, "NoOp"=4060086272, "IO-read_bank0"=3489665024, "IO-write_bank0"=3489660929, "IO-read_bank1"=3506442240, "IO-write_bank1"=3506438145, "DA0-0_LED365"=2684354561, "DA0-1_LED385"=2685403137, "DA0-2_LED440"=2686451713, "DA0-3_LED470"=2687500289, "DA0-4_LED510"=2688548865, "DA0-5_LED550"=2689597441, "DA0-6_LED590"=2690646017, "DA0-7_LED640"=2691694593, "DA1-0_LED-R"=2701131777, "DA1-1_LED-G"=2702180353, "DA1-2_LED-B"=2703228929, "DA1-3_LED-AF"=2704277505, "DA1-4"=2705326081, "DA1-5"=2706374657, "DA1-6"=2707423233, "DA1-7"=2708471809, "DA2-Laser0"=2717908993, "DA2-Laser1"=2718957569, "DA2-Laser2"=2720006145, "DA2-Laser3"=2721054721, "DA2-Laser4"=2722103297, "Analog-read_AD0-0"=2818576384, "Analog-read-store_AD0-0"=2818572290, "IO-delay_bank0"=3489923073, "IO-delay_bank0_fromVar"=3489923075, "read_cam_clock"=3289124864, "store_cam_clock"=3289120770, "read_cam_phase"=3289190400, "store_cam_phase"=3289186306, "store_cam_phase-t"=3289190402, "Read ticks"=4026535936, "Read ticks to var"=4026535938, "Read IP"=4043313152, "Read IP into var"=4043313154, "Set IP from var"=4043309059, "Set IP from var, relative"=4043313155, "branchRel_if_equal"=4043374849, "decrement_branchRel_if_equal"=4043374945, "decrement_branchRel_if_greaterequal"=4043375201, "decrement_branchRel_if_greaterequal_withTicket"=4043379297, "decrement_branchRel_if_smaller"=4043375457, "increment_branchRel_if_smaller"=4043375473, "readVar"=4060090368, "writeVar"=4060086273, "copyVar0_from_var1"=4060086275, "math_addToVariable"=4076863488, "math_addVToVariable"=4076863489, "math_subToVariable"=4076863490, "math_subVToVariable"=4076863491, "math_multToVariable"=4076863492, "math_multvToVariable"=4076863493, "math_divideToVariable"=4076863494, "math_divideVToVariable"=4076863495, "math_modToVariable"=4076863496, "math_modVToVariable"=4076863497, "logic_and"=4093640704, "logic_or"=4093640706, "logic_xor"=4093640708, "bitshift"=4093640712, "set_1Galvo"=101712113, "set_x-Galvo"=102760689, "set_y-Galvo"=103809265, "set_z-Fokus"=104857841, "set_1Galvo_position-only"=101711937, "set_x-Galvo_position-only"=102760513, "set_y-Galvo_position-only"=103809089, "set_z-Fokus_position-only"=104857665, "set_x-Galvo_position-only_ticket"=102764609, "set_y-Galvo_position-only_ticket"=103813185, "set_z-Fokus_position-only_ticket"=104861761, "set_1Galvo_relativ-only"=101712001, "set_x-Galvo_relativ-only"=102760577, "set_y-Galvo_relativ-only"=103809153, "set_z-Fokus_relativ-only"=104857729, "set_1Galvo_speed-only"=101711905, "set_x-Galvo_speed-only"=102760481, "set_y-Galvo_speed-only"=103809057, "set_z-Fokus_speed-only"=104857633, "set_1Galvo_acc-only"=101711889, "set_x-Galvo_acc-only"=102760465, "set_y-Galvo_acc-only"=103809041, "set_z-Fokus_acc-only"=104857617, "read_1Galvo_ticket"=101716032, "read_x-Galvo_ticket"=102764608, "read_y-Galvo_ticket"=103813184, "read_z-Focus_ticket"=104861760, "x-Galvo_pos_fromVar"=102760515, "y-Galvo_pos_fromVar"=103809091, "z-Focus_pos_fromVar"=104857667, "Servo0"=67108865, "Servo0-enable"=68091911, "Servo0-disable"=68091919, "Servo1"=68157441, "Servo1-enable"=69140487, "Servo1-disable"=69140495, "Servo2-enable"=70189063, "Servo2"=69206017, "Servo3-enable"=71237639, "Servo3"=70254593, "x-ssi-init"=202309639, "x-ssi-disable"=202309647, "x-ssi-Bits"=201523201, "x-ssi-Read"=201330688, "x-ssi-ReadToVar"=201326594, "x-ssi-ReadToVar-ticket"=201330690, "y-ssi-init"=203358215, "y-ssi-disable"=203358223, "y-ssi-Bits"=202571777, "y-ssi-Read"=202379264, "y-ssi-ReadToVar"=202375170, "y-ssi-ReadToVat-ticket"=202379266] ("command")
  (unwired) u32 46 ("Delay 10µs")
  w99 = T3 3489660929 items=["read_x-Motor_status_ticket"=17305600, "init_x-Motor"=17760263, "read_x-Motor_absolute_ticket"=16781312, "move_x-Motor_absolute"=16777217, "move_x-Motor_relative"=16842753, "read_y-Motor_status_ticket"=18354176, "init_y-Motor"=18808839, "read_y-Motor_absolute_ticket"=17829888, "move_y-Motor_absolute"=17825793, "move_y-Motor_relative"=17891329, "read_z-Motor_status_ticket"=19402752, "init_z-Motor"=19857415, "stop_z-Motor"=19857423, "start_z-Motor"=19857422, "read_z-Motor_absolute_ticket"=18878464, "move_z-Motor_absolute"=18874369, "move_z-Motor_relative"=18939905, "end_no_ticket"=4027514895, "end_ticket"=4027518991, "IO-read_bank0"=3489665024, "IO-write_bank0"=3489660929, "IO-read_bank1"=3506442240, "IO-write_bank1"=3506438145, "IO-delay_bank0"=3489923073, "IO-delay_bank0_fromVar"=3489923075, "read_cam_clock"=3289124864, "store_cam_clock"=3289120770, "read_cam_phase"=3289190400, "set_cam_deadtime"=3288989697, "set_cam_10uscycles"=3289055233, "set_cam_10uscycles_fromVariable"=3289055235, "calc_cam"=3289317386, "store_cam_Var"=3289251842, "math_addToVariable"=4060086278, "readVar"=4060090368, "writeVar"=4060086273, "copyVar"=4060086276, "decrement_branchRel_if_equal"=4043374945, "decrement_branchRel_if_greaterequal"=4043375201, "decrement_branchRel_if_greaterequal_withTicket"=4043379297, "decrement_branchRel_if_smaller"=4043375457, "increment_branchRel_if_smaller"=4043375473, "set_x-Galvo"=1612710129, "set_y-Galvo"=1613758705, "set_z-Fokus"=1614807281, "set_x-Galvo_position-only"=1612709953, "set_y-Galvo_position-only"=1613758529, "set_z-Fokus_position-only"=1614807105, "set_x-Galvo_position-only_ticket"=1612714049, "set_y-Galvo_position-only_ticket"=1613762625, "set_z-Fokus_position-only_ticket"=1614811201, "read_x-Galvo_ticket"=1612714048, "read_y-Galvo_ticket"=1613762624, "read_z-Focus_ticket"=1614811200, "x-Galvo_pos_fromVar"=1612709955, "y-Galvo_pos_fromVar"=1613758531, "z-Focus_pos_fromVar"=1614807107] ("command")
  w101 = 0  # a off
  w136 = T3 3489660929 items=["read_x-Motor_status_ticket"=17305600, "init_x-Motor"=17760263, "read_x-Motor_absolute_ticket"=16781312, "move_x-Motor_absolute"=16777217, "move_x-Motor_relative"=16842753, "read_y-Motor_status_ticket"=18354176, "init_y-Motor"=18808839, "read_y-Motor_absolute_ticket"=17829888, "move_y-Motor_absolute"=17825793, "move_y-Motor_relative"=17891329, "read_z-Motor_status_ticket"=19402752, "init_z-Motor"=19857415, "stop_z-Motor"=19857423, "start_z-Motor"=19857422, "read_z-Motor_absolute_ticket"=18878464, "move_z-Motor_absolute"=18874369, "move_z-Motor_relative"=18939905, "end_no_ticket"=4027514895, "end_ticket"=4027518991, "IO-read_bank0"=3489665024, "IO-write_bank0"=3489660929, "IO-read_bank1"=3506442240, "IO-write_bank1"=3506438145, "IO-delay_bank0"=3489923073, "IO-delay_bank0_fromVar"=3489923075, "read_cam_clock"=3289124864, "store_cam_clock"=3289120770, "read_cam_phase"=3289190400, "set_cam_deadtime"=3288989697, "set_cam_10uscycles"=3289055233, "set_cam_10uscycles_fromVariable"=3289055235, "calc_cam"=3289317386, "store_cam_Var"=3289251842, "math_addToVariable"=4060086278, "readVar"=4060090368, "writeVar"=4060086273, "copyVar"=4060086276, "decrement_branchRel_if_equal"=4043374945, "decrement_branchRel_if_greaterequal"=4043375201, "decrement_branchRel_if_greaterequal_withTicket"=4043379297, "decrement_branchRel_if_smaller"=4043375457, "increment_branchRel_if_smaller"=4043375473, "set_x-Galvo"=1612710129, "set_y-Galvo"=1613758705, "set_z-Fokus"=1614807281, "set_x-Galvo_position-only"=1612709953, "set_y-Galvo_position-only"=1613758529, "set_z-Fokus_position-only"=1614807105, "set_x-Galvo_position-only_ticket"=1612714049, "set_y-Galvo_position-only_ticket"=1613762625, "set_z-Fokus_position-only_ticket"=1614811201, "read_x-Galvo_ticket"=1612714048, "read_y-Galvo_ticket"=1613762624, "read_z-Focus_ticket"=1614811200, "x-Galvo_pos_fromVar"=1612709955, "y-Galvo_pos_fromVar"=1613758531, "z-Focus_pos_fromVar"=1614807107] ("command")
  w21 = T8 {"Delay 10µs"=0, "command"=4027514895, "P0"=0, "P1"=0, "P2"=0, "P3"=0, "P4"=0, "P5-ticket"=0, "comment"=""} ("Cluster")
  (unwired) T9 [{"Delay 10µs"=0, "command"=3289120770, "P0"=1, "P1"=0, "P2"=0, "P3"=0, "P4"=0, "P5-ticket"=0}]  # startconstants
  w157 = 1  # 1 will be repeated
  w160 = 2  # Var
  w156 = -10  # commands in loop
  w161 = T3 4043379297 items=["read_x-Motor_status_ticket"=17305600, "init_x-Motor"=17760263, "read_x-Motor_absolute_ticket"=16781312, "move_x-Motor_absolute"=16777217, "move_x-Motor_relative"=16842753, "read_x-Motor_speed"=16977920, "set_x-Motor_speed"=16973825, "read_y-Motor_status_ticket"=18354176, "init_y-Motor"=18808839, "read_y-Motor_absolute_ticket"=17829888, "move_y-Motor_absolute"=17825793, "move_y-Motor_relative"=17891329, "read_y-Motor_speed"=18026496, "set_y-Motor_speed"=18022401, "read_z-Motor_status_ticket"=19402752, "init_z-Motor"=19857415, "stop_z-Motor"=19857423, "start_z-Motor"=19857422, "read_z-Motor_absolute_ticket"=18878464, "move_z-Motor_absolute"=18874369, "move_z-Motor_relative"=18939905, "read_Objective_status_ticket"=20451328, "init_Objective"=20905991, "read_Objective_absolute_ticket"=19927040, "move_Objective_absolute"=19922945, "move_Objective_relative"=19988481, "read_Objective-Motor_speed"=20123648, "set_Objective-Motor_speed"=20119553, "read_Filter_status_ticket"=21499904, "init_Filter"=21954567, "read_Filter_absolute_ticket"=20975616, "move_Filter_absolute"=20971521, "move_Filter_relative"=21037057, "read_Filter-Motor_speed"=21172224, "set_Filter-Motor_speed"=21168129, "read_Trans-Rad_status_ticket"=22548480, "init_Trans-Rad"=23003143, "read_Trans-Rad_absolute_ticket"=22024192, "move_Trans-Rad_absolute"=22020097, "move_Trans-Rad_relative"=22085633, "read_Trans-Motor_speed"=22220800, "set_Trans-Motor_speed"=22216705, "read_FRET_status_ticket"=23597056, "init_FRET"=24051719, "read_FRET_absolute_ticket"=23072768, "move_FRET_absolute"=23068673, "move_FRET_relative"=23134209, "read_FRET-Motor_speed"=23269376, "set_FRET-Motor_speed"=23265281, "read_SI-Rad_status_ticket"=24645632, "init_SI-Rad"=25100295, "read_SI-Rad_absolute_ticket"=24121344, "move_SI-Rad_absolute"=24117249, "move_SI-Rad_relative"=24182785, "read_SI-Rad_speed"=24317952, "set_SI-Rad_speed"=24313857, "end_no_ticket"=4027514895, "end_ticket"=4027518991, "IO-read_bank0"=3489665024, "IO-write_bank0"=3489660929, "IO-read_bank1"=3506442240, "IO-write_bank1"=3506438145, "DA0-0_LED365"=2684354561, "DA0-1_LED385"=2685403137, "DA0-2_LED440"=2686451713, "DA0-3_LED470"=2687500289, "DA0-4_LED510"=2688548865, "DA0-5_LED550"=2689597441, "DA0-6_LED590"=2690646017, "DA0-7_LED640"=2691694593, "DA1-0_LED-R"=2701131777, "DA1-1_LED-G"=2702180353, "DA1-2_LED-B"=2703228929, "DA1-3_LED-AF"=2704277505, "DA1-4"=2705326081, "DA1-5"=2706374657, "DA1-6"=2707423233, "DA1-7"=2708471809, "DA2-Laser0"=2717908993, "DA2-Laser1"=2718957569, "DA2-Laser2"=2720006145, "DA2-Laser3"=2721054721, "DA2-Laser4"=2722103297, "Analog-read_AD0-0"=2818576384, "Analog-read-store_AD0-0"=2818572290, "IO-delay_bank0"=3489923073, "IO-delay_bank0_fromVar"=3489923075, "read_cam_clock"=3289124864, "store_cam_clock"=3289120770, "read_cam_phase"=3289190400, "store_cam_phase"=3289190402, "Read ticks"=4027518976, "Read ticks to var"=4027518978, "Read IP"=4043313152, "Read IP into var"=4043313154, "Set IP from var"=4043309059, "Set IP from var, relative"=4043313155, "decrement_branchRel_if_equal"=4043374945, "decrement_branchRel_if_greaterequal"=4043375201, "decrement_branchRel_if_greaterequal_withTicket"=4043379297, "decrement_branchRel_if_smaller"=4043375457, "increment_branchRel_if_smaller"=4043375473, "readVar"=4060090368, "writeVar"=4060086273, "readVar_and_copy_to_var2"=4060086275, "loadVar2_andcopy_var1"=4060086276, "math_addToVariable"=4076863488, "math_addVToVariable"=4076863489, "math_subToVariable"=4076863490, "math_subVToVariable"=4076863491, "math_multToVariable"=4076863492, "math_multvToVariable"=4076863493, "math_divideToVariable"=4076863494, "math_divideVToVariable"=4076863495, "math_modToVariable"=4076863496, "math_modVToVariable"=4076863497, "logic_and"=4093640704, "logic_or"=4093640706, "logic_xor"=4093640708, "set_1Galvo"=101712113, "set_x-Galvo"=102760689, "set_y-Galvo"=103809265, "set_z-Fokus"=104857841, "set_1Galvo_position-only"=101711937, "set_x-Galvo_position-only"=102760513, "set_y-Galvo_position-only"=103809089, "set_z-Fokus_position-only"=104857665, "set_x-Galvo_position-only_ticket"=102764609, "set_y-Galvo_position-only_ticket"=103813185, "set_z-Fokus_position-only_ticket"=104861761, "set_x-Galvo_relativ-only"=102760577, "set_y-Galvo_relativ-only"=103809153, "set_z-Fokus_relativ-only"=104857729, "set_x-Galvo_speed-only"=102760481, "set_y-Galvo_speed-only"=103809057, "set_z-Fokus_speed-only"=104857633, "read_1Galvo_ticket"=101716032, "read_x-Galvo_ticket"=102764608, "read_y-Galvo_ticket"=103813184, "read_z-Focus_ticket"=104861760, "x-Galvo_pos_fromVar"=102760515, "y-Galvo_pos_fromVar"=103809091, "z-Focus_pos_fromVar"=104857667, "Servo0"=67108865, "Servo0-enable"=68091911, "Servo0-disable"=68091919, "Servo1"=68157441, "Servo1-enable"=69140487, "Servo1-disable"=69140495, "EnablePower0-SM"=2148466695, "DisablePower0-SM"=2148466703, "EnablePower1-Thermo1"=2149515271, "DisablePower1-Thermo1"=2149515279, "EnablePower2-Cam"=2150563847, "DisablePower2-Cam"=2150563855, "EnablePower3-Thermo2"=2151612423, "DisablePower3-Thermo2"=2151612431, "EnablePower4-Laser0"=2152660999, "DisablePower4-Laser0"=2152661007, "EnablePower5"=2153709575, "DisablePower5"=2153709583, "EnablePower6-Laser1"=2154758151, "DisablePower6-Laser1"=2154758159, "EnablePower7-SAM"=2155806727, "DisablePower7-SAM"=2155806735, "EnablePower8-Laser2"=2156855303, "DisablePower8-Laser2"=2156855311, "EnablePower9-TSM"=2157903879, "DisablePower9-TSM"=2157903887, "EnablePower10-Laser3"=2158952455, "DisablePower10-Laser3"=2158952463, "EnablePower11-Servo"=2160001031, "DisablePower11-Servo"=2160001039, "EnablePower12-Laser4"=2161049607, "DisablePower12-Laser4"=2161049615, "EnableSMPower2-DCC22"=2167341063, "DisableSMPower2-DCC22"=2167341071, "EnableSMPower3-6220"=2168389639, "DisableSMPower3-6220"=2168389647, "EnableSMPower4-6210"=2169438215, "DisableSMPower4-6210"=2169438223] ("command")
  w162 = u32 2  # 2*0.5 turntimes
  w23 = 5 ("P0")
  w168 = T3 3489660929 items=["read_x-Motor_status_ticket"=17305600, "init_x-Motor"=17760263, "read_x-Motor_absolute_ticket"=16781312, "move_x-Motor_absolute"=16777217, "move_x-Motor_relative"=16842753, "read_y-Motor_status_ticket"=18354176, "init_y-Motor"=18808839, "read_y-Motor_absolute_ticket"=17829888, "move_y-Motor_absolute"=17825793, "move_y-Motor_relative"=17891329, "read_z-Motor_status_ticket"=19402752, "init_z-Motor"=19857415, "stop_z-Motor"=19857423, "start_z-Motor"=19857422, "read_z-Motor_absolute_ticket"=18878464, "move_z-Motor_absolute"=18874369, "move_z-Motor_relative"=18939905, "end_no_ticket"=4027514895, "end_ticket"=4027518991, "IO-read_bank0"=3489665024, "IO-write_bank0"=3489660929, "IO-read_bank1"=3506442240, "IO-write_bank1"=3506438145, "IO-delay_bank0"=3489923073, "IO-delay_bank0_fromVar"=3489923075, "read_cam_clock"=3289124864, "store_cam_clock"=3289120770, "read_cam_phase"=3289190400, "set_cam_deadtime"=3288989697, "set_cam_10uscycles"=3289055233, "set_cam_10uscycles_fromVariable"=3289055235, "calc_cam"=3289317386, "store_cam_Var"=3289251842, "math_addToVariable"=4060086278, "readVar"=4060090368, "writeVar"=4060086273, "copyVar"=4060086276, "decrement_branchRel_if_equal"=4043374945, "decrement_branchRel_if_greaterequal"=4043375201, "decrement_branchRel_if_greaterequal_withTicket"=4043379297, "decrement_branchRel_if_smaller"=4043375457, "increment_branchRel_if_smaller"=4043375473, "set_x-Galvo"=1612710129, "set_y-Galvo"=1613758705, "set_z-Fokus"=1614807281, "set_x-Galvo_position-only"=1612709953, "set_y-Galvo_position-only"=1613758529, "set_z-Fokus_position-only"=1614807105, "set_x-Galvo_position-only_ticket"=1612714049, "set_y-Galvo_position-only_ticket"=1613762625, "set_z-Fokus_position-only_ticket"=1614811201, "read_x-Galvo_ticket"=1612714048, "read_y-Galvo_ticket"=1613762624, "read_z-Focus_ticket"=1614811200, "x-Galvo_pos_fromVar"=1612709955, "y-Galvo_pos_fromVar"=1613758531, "z-Focus_pos_fromVar"=1614807107] ("command")
  w183 = 2  # Var2 linecounter (subframe)
  w185 = T3 4060086273 items=["read_x-Motor_status_ticket"=17305600, "init_x-Motor"=17760263, "read_x-Motor_absolute_ticket"=16781312, "move_x-Motor_absolute"=16777217, "move_x-Motor_relative"=16842753, "read_x-Motor_speed"=16977920, "set_x-Motor_speed"=16973825, "read_y-Motor_status_ticket"=18354176, "init_y-Motor"=18808839, "read_y-Motor_absolute_ticket"=17829888, "move_y-Motor_absolute"=17825793, "move_y-Motor_relative"=17891329, "read_y-Motor_speed"=18026496, "set_y-Motor_speed"=18022401, "read_z-Motor_status_ticket"=19402752, "init_z-Motor"=19857415, "stop_z-Motor"=19857423, "start_z-Motor"=19857422, "read_z-Motor_absolute_ticket"=18878464, "move_z-Motor_absolute"=18874369, "move_z-Motor_relative"=18939905, "read_Objective_status_ticket"=20451328, "init_Objective"=20905991, "read_Objective_absolute_ticket"=19927040, "move_Objective_absolute"=19922945, "move_Objective_relative"=19988481, "read_Objective-Motor_speed"=20123648, "set_Objective-Motor_speed"=20119553, "read_Filter_status_ticket"=21499904, "init_Filter"=21954567, "read_Filter_absolute_ticket"=20975616, "move_Filter_absolute"=20971521, "move_Filter_relative"=21037057, "read_Filter-Motor_speed"=21172224, "set_Filter-Motor_speed"=21168129, "read_Trans-Rad_status_ticket"=22548480, "init_Trans-Rad"=23003143, "read_Trans-Rad_absolute_ticket"=22024192, "move_Trans-Rad_absolute"=22020097, "move_Trans-Rad_relative"=22085633, "read_Trans-Motor_speed"=22220800, "set_Trans-Motor_speed"=22216705, "read_FRET_status_ticket"=23597056, "init_FRET"=24051719, "read_FRET_absolute_ticket"=23072768, "move_FRET_absolute"=23068673, "move_FRET_relative"=23134209, "read_FRET-Motor_speed"=23269376, "set_FRET-Motor_speed"=23265281, "read_SI-Rad_status_ticket"=24645632, "init_SI-Rad"=25100295, "read_SI-Rad_absolute_ticket"=24121344, "move_SI-Rad_absolute"=24117249, "move_SI-Rad_relative"=24182785, "read_SI-Rad_speed"=24317952, "set_SI-Rad_speed"=24313857, "end_no_ticket"=4027514895, "end_ticket"=4027518991, "IO-read_bank0"=3489665024, "IO-write_bank0"=3489660929, "IO-read_bank1"=3506442240, "IO-write_bank1"=3506438145, "DA0-0_LED365"=2684354561, "DA0-1_LED385"=2685403137, "DA0-2_LED440"=2686451713, "DA0-3_LED470"=2687500289, "DA0-4_LED510"=2688548865, "DA0-5_LED550"=2689597441, "DA0-6_LED590"=2690646017, "DA0-7_LED640"=2691694593, "DA1-0_LED-R"=2701131777, "DA1-1_LED-G"=2702180353, "DA1-2_LED-B"=2703228929, "DA1-3_LED-AF"=2704277505, "DA1-4"=2705326081, "DA1-5"=2706374657, "DA1-6"=2707423233, "DA1-7"=2708471809, "DA2-Laser0"=2717908993, "DA2-Laser1"=2718957569, "DA2-Laser2"=2720006145, "DA2-Laser3"=2721054721, "DA2-Laser4"=2722103297, "Analog-read_AD0-0"=2818576384, "Analog-read-store_AD0-0"=2818572290, "IO-delay_bank0"=3489923073, "IO-delay_bank0_fromVar"=3489923075, "read_cam_clock"=3289124864, "store_cam_clock"=3289120770, "read_cam_phase"=3289190400, "store_cam_phase"=3289190402, "Read ticks"=4027518976, "Read ticks to var"=4027518978, "Read IP"=4043313152, "Read IP into var"=4043313154, "Set IP from var"=4043309059, "Set IP from var, relative"=4043313155, "decrement_branchRel_if_equal"=4043374945, "decrement_branchRel_if_greaterequal"=4043375201, "decrement_branchRel_if_greaterequal_withTicket"=4043379297, "decrement_branchRel_if_smaller"=4043375457, "increment_branchRel_if_smaller"=4043375473, "readVar"=4060090368, "writeVar"=4060086273, "readVar_and_copy_to_var2"=4060086275, "loadVar2_andcopy_var1"=4060086276, "math_addToVariable"=4076863488, "math_addVToVariable"=4076863489, "math_subToVariable"=4076863490, "math_subVToVariable"=4076863491, "math_multToVariable"=4076863492, "math_multvToVariable"=4076863493, "math_divideToVariable"=4076863494, "math_divideVToVariable"=4076863495, "math_modToVariable"=4076863496, "math_modVToVariable"=4076863497, "logic_and"=4093640704, "logic_or"=4093640706, "logic_xor"=4093640708, "set_1Galvo"=101712113, "set_x-Galvo"=102760689, "set_y-Galvo"=103809265, "set_z-Fokus"=104857841, "set_1Galvo_position-only"=101711937, "set_x-Galvo_position-only"=102760513, "set_y-Galvo_position-only"=103809089, "set_z-Fokus_position-only"=104857665, "set_x-Galvo_position-only_ticket"=102764609, "set_y-Galvo_position-only_ticket"=103813185, "set_z-Fokus_position-only_ticket"=104861761, "set_x-Galvo_relativ-only"=102760577, "set_y-Galvo_relativ-only"=103809153, "set_z-Fokus_relativ-only"=104857729, "set_x-Galvo_speed-only"=102760481, "set_y-Galvo_speed-only"=103809057, "set_z-Fokus_speed-only"=104857633, "read_1Galvo_ticket"=101716032, "read_x-Galvo_ticket"=102764608, "read_y-Galvo_ticket"=103813184, "read_z-Focus_ticket"=104861760, "x-Galvo_pos_fromVar"=102760515, "y-Galvo_pos_fromVar"=103809091, "z-Focus_pos_fromVar"=104857667, "Servo0"=67108865, "Servo0-enable"=68091911, "Servo0-disable"=68091919, "Servo1"=68157441, "Servo1-enable"=69140487, "Servo1-disable"=69140495, "EnablePower0-SM"=2148466695, "DisablePower0-SM"=2148466703, "EnablePower1-Thermo1"=2149515271, "DisablePower1-Thermo1"=2149515279, "EnablePower2-Cam"=2150563847, "DisablePower2-Cam"=2150563855, "EnablePower3-Thermo2"=2151612423, "DisablePower3-Thermo2"=2151612431, "EnablePower4-Laser0"=2152660999, "DisablePower4-Laser0"=2152661007, "EnablePower5"=2153709575, "DisablePower5"=2153709583, "EnablePower6-Laser1"=2154758151, "DisablePower6-Laser1"=2154758159, "EnablePower7-SAM"=2155806727, "DisablePower7-SAM"=2155806735, "EnablePower8-Laser2"=2156855303, "DisablePower8-Laser2"=2156855311, "EnablePower9-TSM"=2157903879, "DisablePower9-TSM"=2157903887, "EnablePower10-Laser3"=2158952455, "DisablePower10-Laser3"=2158952463, "EnablePower11-Servo"=2160001031, "DisablePower11-Servo"=2160001039, "EnablePower12-Laser4"=2161049607, "DisablePower12-Laser4"=2161049615, "EnableSMPower2-DCC22"=2167341063, "DisableSMPower2-DCC22"=2167341071, "EnableSMPower3-6220"=2168389639, "DisableSMPower3-6220"=2168389647, "EnableSMPower4-6210"=2169438215, "DisableSMPower4-6210"=2169438223] ("command")
  w193 = 10.0  # µs
  w199 = 123456789.0  # no speedlimit
  w207 = 1  # 1 will be repeated
  w209 = 3  # Var
  w210 = -6  # commands in loop
  w211 = T3 4043379297 items=["read_x-Motor_status_ticket"=17305600, "init_x-Motor"=17760263, "read_x-Motor_absolute_ticket"=16781312, "move_x-Motor_absolute"=16777217, "move_x-Motor_relative"=16842753, "read_x-Motor_speed"=16977920, "set_x-Motor_speed"=16973825, "read_y-Motor_status_ticket"=18354176, "init_y-Motor"=18808839, "read_y-Motor_absolute_ticket"=17829888, "move_y-Motor_absolute"=17825793, "move_y-Motor_relative"=17891329, "read_y-Motor_speed"=18026496, "set_y-Motor_speed"=18022401, "read_z-Motor_status_ticket"=19402752, "init_z-Motor"=19857415, "stop_z-Motor"=19857423, "start_z-Motor"=19857422, "read_z-Motor_absolute_ticket"=18878464, "move_z-Motor_absolute"=18874369, "move_z-Motor_relative"=18939905, "read_Objective_status_ticket"=20451328, "init_Objective"=20905991, "read_Objective_absolute_ticket"=19927040, "move_Objective_absolute"=19922945, "move_Objective_relative"=19988481, "read_Objective-Motor_speed"=20123648, "set_Objective-Motor_speed"=20119553, "read_Filter_status_ticket"=21499904, "init_Filter"=21954567, "read_Filter_absolute_ticket"=20975616, "move_Filter_absolute"=20971521, "move_Filter_relative"=21037057, "read_Filter-Motor_speed"=21172224, "set_Filter-Motor_speed"=21168129, "read_Trans-Rad_status_ticket"=22548480, "init_Trans-Rad"=23003143, "read_Trans-Rad_absolute_ticket"=22024192, "move_Trans-Rad_absolute"=22020097, "move_Trans-Rad_relative"=22085633, "read_Trans-Motor_speed"=22220800, "set_Trans-Motor_speed"=22216705, "read_FRET_status_ticket"=23597056, "init_FRET"=24051719, "read_FRET_absolute_ticket"=23072768, "move_FRET_absolute"=23068673, "move_FRET_relative"=23134209, "read_FRET-Motor_speed"=23269376, "set_FRET-Motor_speed"=23265281, "read_SI-Rad_status_ticket"=24645632, "init_SI-Rad"=25100295, "read_SI-Rad_absolute_ticket"=24121344, "move_SI-Rad_absolute"=24117249, "move_SI-Rad_relative"=24182785, "read_SI-Rad_speed"=24317952, "set_SI-Rad_speed"=24313857, "end_no_ticket"=4027514895, "end_ticket"=4027518991, "IO-read_bank0"=3489665024, "IO-write_bank0"=3489660929, "IO-read_bank1"=3506442240, "IO-write_bank1"=3506438145, "DA0-0_LED365"=2684354561, "DA0-1_LED385"=2685403137, "DA0-2_LED440"=2686451713, "DA0-3_LED470"=2687500289, "DA0-4_LED510"=2688548865, "DA0-5_LED550"=2689597441, "DA0-6_LED590"=2690646017, "DA0-7_LED640"=2691694593, "DA1-0_LED-R"=2701131777, "DA1-1_LED-G"=2702180353, "DA1-2_LED-B"=2703228929, "DA1-3_LED-AF"=2704277505, "DA1-4"=2705326081, "DA1-5"=2706374657, "DA1-6"=2707423233, "DA1-7"=2708471809, "DA2-Laser0"=2717908993, "DA2-Laser1"=2718957569, "DA2-Laser2"=2720006145, "DA2-Laser3"=2721054721, "DA2-Laser4"=2722103297, "Analog-read_AD0-0"=2818576384, "Analog-read-store_AD0-0"=2818572290, "IO-delay_bank0"=3489923073, "IO-delay_bank0_fromVar"=3489923075, "read_cam_clock"=3289124864, "store_cam_clock"=3289120770, "read_cam_phase"=3289190400, "store_cam_phase"=3289190402, "Read ticks"=4027518976, "Read ticks to var"=4027518978, "Read IP"=4043313152, "Read IP into var"=4043313154, "Set IP from var"=4043309059, "Set IP from var, relative"=4043313155, "decrement_branchRel_if_equal"=4043374945, "decrement_branchRel_if_greaterequal"=4043375201, "decrement_branchRel_if_greaterequal_withTicket"=4043379297, "decrement_branchRel_if_smaller"=4043375457, "increment_branchRel_if_smaller"=4043375473, "readVar"=4060090368, "writeVar"=4060086273, "readVar_and_copy_to_var2"=4060086275, "loadVar2_andcopy_var1"=4060086276, "math_addToVariable"=4076863488, "math_addVToVariable"=4076863489, "math_subToVariable"=4076863490, "math_subVToVariable"=4076863491, "math_multToVariable"=4076863492, "math_multvToVariable"=4076863493, "math_divideToVariable"=4076863494, "math_divideVToVariable"=4076863495, "math_modToVariable"=4076863496, "math_modVToVariable"=4076863497, "logic_and"=4093640704, "logic_or"=4093640706, "logic_xor"=4093640708, "set_1Galvo"=101712113, "set_x-Galvo"=102760689, "set_y-Galvo"=103809265, "set_z-Fokus"=104857841, "set_1Galvo_position-only"=101711937, "set_x-Galvo_position-only"=102760513, "set_y-Galvo_position-only"=103809089, "set_z-Fokus_position-only"=104857665, "set_x-Galvo_position-only_ticket"=102764609, "set_y-Galvo_position-only_ticket"=103813185, "set_z-Fokus_position-only_ticket"=104861761, "set_x-Galvo_relativ-only"=102760577, "set_y-Galvo_relativ-only"=103809153, "set_z-Fokus_relativ-only"=104857729, "set_x-Galvo_speed-only"=102760481, "set_y-Galvo_speed-only"=103809057, "set_z-Fokus_speed-only"=104857633, "read_1Galvo_ticket"=101716032, "read_x-Galvo_ticket"=102764608, "read_y-Galvo_ticket"=103813184, "read_z-Focus_ticket"=104861760, "x-Galvo_pos_fromVar"=102760515, "y-Galvo_pos_fromVar"=103809091, "z-Focus_pos_fromVar"=104857667, "Servo0"=67108865, "Servo0-enable"=68091911, "Servo0-disable"=68091919, "Servo1"=68157441, "Servo1-enable"=69140487, "Servo1-disable"=69140495, "EnablePower0-SM"=2148466695, "DisablePower0-SM"=2148466703, "EnablePower1-Thermo1"=2149515271, "DisablePower1-Thermo1"=2149515279, "EnablePower2-Cam"=2150563847, "DisablePower2-Cam"=2150563855, "EnablePower3-Thermo2"=2151612423, "DisablePower3-Thermo2"=2151612431, "EnablePower4-Laser0"=2152660999, "DisablePower4-Laser0"=2152661007, "EnablePower5"=2153709575, "DisablePower5"=2153709583, "EnablePower6-Laser1"=2154758151, "DisablePower6-Laser1"=2154758159, "EnablePower7-SAM"=2155806727, "DisablePower7-SAM"=2155806735, "EnablePower8-Laser2"=2156855303, "DisablePower8-Laser2"=2156855311, "EnablePower9-TSM"=2157903879, "DisablePower9-TSM"=2157903887, "EnablePower10-Laser3"=2158952455, "DisablePower10-Laser3"=2158952463, "EnablePower11-Servo"=2160001031, "DisablePower11-Servo"=2160001039, "EnablePower12-Laser4"=2161049607, "DisablePower12-Laser4"=2161049615, "EnableSMPower2-DCC22"=2167341063, "DisableSMPower2-DCC22"=2167341071, "EnableSMPower3-6220"=2168389639, "DisableSMPower3-6220"=2168389647, "EnableSMPower4-6210"=2169438215, "DisableSMPower4-6210"=2169438223] ("command")
  w212 = 3  # Var3  framecounter
  w214 = T3 4060086273 items=["read_x-Motor_status_ticket"=17305600, "init_x-Motor"=17760263, "read_x-Motor_absolute_ticket"=16781312, "move_x-Motor_absolute"=16777217, "move_x-Motor_relative"=16842753, "read_x-Motor_speed"=16977920, "set_x-Motor_speed"=16973825, "read_y-Motor_status_ticket"=18354176, "init_y-Motor"=18808839, "read_y-Motor_absolute_ticket"=17829888, "move_y-Motor_absolute"=17825793, "move_y-Motor_relative"=17891329, "read_y-Motor_speed"=18026496, "set_y-Motor_speed"=18022401, "read_z-Motor_status_ticket"=19402752, "init_z-Motor"=19857415, "stop_z-Motor"=19857423, "start_z-Motor"=19857422, "read_z-Motor_absolute_ticket"=18878464, "move_z-Motor_absolute"=18874369, "move_z-Motor_relative"=18939905, "read_Objective_status_ticket"=20451328, "init_Objective"=20905991, "read_Objective_absolute_ticket"=19927040, "move_Objective_absolute"=19922945, "move_Objective_relative"=19988481, "read_Objective-Motor_speed"=20123648, "set_Objective-Motor_speed"=20119553, "read_Filter_status_ticket"=21499904, "init_Filter"=21954567, "read_Filter_absolute_ticket"=20975616, "move_Filter_absolute"=20971521, "move_Filter_relative"=21037057, "read_Filter-Motor_speed"=21172224, "set_Filter-Motor_speed"=21168129, "read_Trans-Rad_status_ticket"=22548480, "init_Trans-Rad"=23003143, "read_Trans-Rad_absolute_ticket"=22024192, "move_Trans-Rad_absolute"=22020097, "move_Trans-Rad_relative"=22085633, "read_Trans-Motor_speed"=22220800, "set_Trans-Motor_speed"=22216705, "read_FRET_status_ticket"=23597056, "init_FRET"=24051719, "read_FRET_absolute_ticket"=23072768, "move_FRET_absolute"=23068673, "move_FRET_relative"=23134209, "read_FRET-Motor_speed"=23269376, "set_FRET-Motor_speed"=23265281, "read_SI-Rad_status_ticket"=24645632, "init_SI-Rad"=25100295, "read_SI-Rad_absolute_ticket"=24121344, "move_SI-Rad_absolute"=24117249, "move_SI-Rad_relative"=24182785, "read_SI-Rad_speed"=24317952, "set_SI-Rad_speed"=24313857, "end_no_ticket"=4027514895, "end_ticket"=4027518991, "IO-read_bank0"=3489665024, "IO-write_bank0"=3489660929, "IO-read_bank1"=3506442240, "IO-write_bank1"=3506438145, "DA0-0_LED365"=2684354561, "DA0-1_LED385"=2685403137, "DA0-2_LED440"=2686451713, "DA0-3_LED470"=2687500289, "DA0-4_LED510"=2688548865, "DA0-5_LED550"=2689597441, "DA0-6_LED590"=2690646017, "DA0-7_LED640"=2691694593, "DA1-0_LED-R"=2701131777, "DA1-1_LED-G"=2702180353, "DA1-2_LED-B"=2703228929, "DA1-3_LED-AF"=2704277505, "DA1-4"=2705326081, "DA1-5"=2706374657, "DA1-6"=2707423233, "DA1-7"=2708471809, "DA2-Laser0"=2717908993, "DA2-Laser1"=2718957569, "DA2-Laser2"=2720006145, "DA2-Laser3"=2721054721, "DA2-Laser4"=2722103297, "Analog-read_AD0-0"=2818576384, "Analog-read-store_AD0-0"=2818572290, "IO-delay_bank0"=3489923073, "IO-delay_bank0_fromVar"=3489923075, "read_cam_clock"=3289124864, "store_cam_clock"=3289120770, "read_cam_phase"=3289190400, "store_cam_phase"=3289190402, "Read ticks"=4027518976, "Read ticks to var"=4027518978, "Read IP"=4043313152, "Read IP into var"=4043313154, "Set IP from var"=4043309059, "Set IP from var, relative"=4043313155, "decrement_branchRel_if_equal"=4043374945, "decrement_branchRel_if_greaterequal"=4043375201, "decrement_branchRel_if_greaterequal_withTicket"=4043379297, "decrement_branchRel_if_smaller"=4043375457, "increment_branchRel_if_smaller"=4043375473, "readVar"=4060090368, "writeVar"=4060086273, "readVar_and_copy_to_var2"=4060086275, "loadVar2_andcopy_var1"=4060086276, "math_addToVariable"=4076863488, "math_addVToVariable"=4076863489, "math_subToVariable"=4076863490, "math_subVToVariable"=4076863491, "math_multToVariable"=4076863492, "math_multvToVariable"=4076863493, "math_divideToVariable"=4076863494, "math_divideVToVariable"=4076863495, "math_modToVariable"=4076863496, "math_modVToVariable"=4076863497, "logic_and"=4093640704, "logic_or"=4093640706, "logic_xor"=4093640708, "set_1Galvo"=101712113, "set_x-Galvo"=102760689, "set_y-Galvo"=103809265, "set_z-Fokus"=104857841, "set_1Galvo_position-only"=101711937, "set_x-Galvo_position-only"=102760513, "set_y-Galvo_position-only"=103809089, "set_z-Fokus_position-only"=104857665, "set_x-Galvo_position-only_ticket"=102764609, "set_y-Galvo_position-only_ticket"=103813185, "set_z-Fokus_position-only_ticket"=104861761, "set_x-Galvo_relativ-only"=102760577, "set_y-Galvo_relativ-only"=103809153, "set_z-Fokus_relativ-only"=104857729, "set_x-Galvo_speed-only"=102760481, "set_y-Galvo_speed-only"=103809057, "set_z-Fokus_speed-only"=104857633, "read_1Galvo_ticket"=101716032, "read_x-Galvo_ticket"=102764608, "read_y-Galvo_ticket"=103813184, "read_z-Focus_ticket"=104861760, "x-Galvo_pos_fromVar"=102760515, "y-Galvo_pos_fromVar"=103809091, "z-Focus_pos_fromVar"=104857667, "Servo0"=67108865, "Servo0-enable"=68091911, "Servo0-disable"=68091919, "Servo1"=68157441, "Servo1-enable"=69140487, "Servo1-disable"=69140495, "EnablePower0-SM"=2148466695, "DisablePower0-SM"=2148466703, "EnablePower1-Thermo1"=2149515271, "DisablePower1-Thermo1"=2149515279, "EnablePower2-Cam"=2150563847, "DisablePower2-Cam"=2150563855, "EnablePower3-Thermo2"=2151612423, "DisablePower3-Thermo2"=2151612431, "EnablePower4-Laser0"=2152660999, "DisablePower4-Laser0"=2152661007, "EnablePower5"=2153709575, "DisablePower5"=2153709583, "EnablePower6-Laser1"=2154758151, "DisablePower6-Laser1"=2154758159, "EnablePower7-SAM"=2155806727, "DisablePower7-SAM"=2155806735, "EnablePower8-Laser2"=2156855303, "DisablePower8-Laser2"=2156855311, "EnablePower9-TSM"=2157903879, "DisablePower9-TSM"=2157903887, "EnablePower10-Laser3"=2158952455, "DisablePower10-Laser3"=2158952463, "EnablePower11-Servo"=2160001031, "DisablePower11-Servo"=2160001039, "EnablePower12-Laser4"=2161049607, "DisablePower12-Laser4"=2161049615, "EnableSMPower2-DCC22"=2167341063, "DisableSMPower2-DCC22"=2167341071, "EnableSMPower3-6220"=2168389639, "DisableSMPower3-6220"=2168389647, "EnableSMPower4-6210"=2169438215, "DisableSMPower4-6210"=2169438223] ("command")
  w225 = T3 4027518991 items=["read_x-Motor_status_ticket"=17305600, "init_x-Motor"=17760263, "read_x-Motor_absolute_ticket"=16781312, "move_x-Motor_absolute"=16777217, "move_x-Motor_relative"=16842753, "read_y-Motor_status_ticket"=18354176, "init_y-Motor"=18808839, "read_y-Motor_absolute_ticket"=17829888, "move_y-Motor_absolute"=17825793, "move_y-Motor_relative"=17891329, "read_z-Motor_status_ticket"=19402752, "init_z-Motor"=19857415, "stop_z-Motor"=19857423, "start_z-Motor"=19857422, "read_z-Motor_absolute_ticket"=18878464, "move_z-Motor_absolute"=18874369, "move_z-Motor_relative"=18939905, "end_no_ticket"=4027514895, "end_ticket"=4027518991, "IO-read_bank0"=3489665024, "IO-write_bank0"=3489660929, "IO-read_bank1"=3506442240, "IO-write_bank1"=3506438145, "IO-delay_bank0"=3489923073, "IO-delay_bank0_fromVar"=3489923075, "read_cam_clock"=3289124864, "store_cam_clock"=3289120770, "read_cam_phase"=3289190400, "set_cam_deadtime"=3288989697, "set_cam_10uscycles"=3289055233, "set_cam_10uscycles_fromVariable"=3289055235, "calc_cam"=3289317386, "store_cam_Var"=3289251842, "math_addToVariable"=4060086278, "readVar"=4060090368, "writeVar"=4060086273, "copyVar"=4060086276, "decrement_branchRel_if_equal"=4043374945, "decrement_branchRel_if_greaterequal"=4043375201, "decrement_branchRel_if_greaterequal_withTicket"=4043379297, "decrement_branchRel_if_smaller"=4043375457, "increment_branchRel_if_smaller"=4043375473, "set_x-Galvo"=1612710129, "set_y-Galvo"=1613758705, "set_z-Fokus"=1614807281, "set_x-Galvo_position-only"=1612709953, "set_y-Galvo_position-only"=1613758529, "set_z-Fokus_position-only"=1614807105, "set_x-Galvo_position-only_ticket"=1612714049, "set_y-Galvo_position-only_ticket"=1613762625, "set_z-Fokus_position-only_ticket"=1614811201, "read_x-Galvo_ticket"=1612714048, "read_y-Galvo_ticket"=1613762624, "read_z-Focus_ticket"=1614811200, "x-Galvo_pos_fromVar"=1612709955, "y-Galvo_pos_fromVar"=1613758531, "z-Focus_pos_fromVar"=1614807107] ("command")
  # "stopp all galvo1"
  # "hier kein n+1: 8Pfosten 7Felder"
  # "??? check\netwas zu viel"
  # "hmm 99 zu weit\nwird bei vielen t besser"
  # "??? check\netwas zu viel"
  # "prepare next z\nstopp x\nreturn ch1"
  # "give some time for strat jump"
  # "linear weiter, prepare for jump"
  # "wieder bremsen"
  # "laser aus ~116 nach turn start\nmitten im turn ist OK"
  # "1. rampe"
  # "stopp all, goto blanking"
  # "linear frame here\nloop point"
  # "P order is rel,abs,inc,incinc!"
  # "bis hier etwa OK"
  # "PhaseTurn"
  # "ende linear\nparabolic galvo turn"
  # "galvo start pos, jump ok ~0"
  # "wobbler start pos, sorry jump! speed off"
  # "start position\n0.5 RS above"
  # "a parabolic move:\nx=a/2 *t(t-1)+v*t"
  n1 = Unbundle By Name("Constants") -> ("RS height- Pix"=w152:u16, "GalvoX-Blanking"=w218:dbl, "Wobbel-total"=w155:dbl, "min turn ticks"=w54:dbl, "WobbelAccel"=w196:dbl, "galvoxAccel"=w195:dbl, "Camera-StartLine"=w145:i32, "Camera-Endline"=w146:u32, "galvox-Line0"=w190:i16, "galvox-count/pix"=w149:dbl, "SCMOS-LineSpeed [10µs]"=w141:dbl, "SM_ticks"=w82:u32, "z-delay-ticks"=w35:u32)
  n2 = Unbundle By Name("User") -> ("z-distance_motorunits"=w66:i32, "#planes"=w200:u16, "NoOfPhaseImages"=w151:u16)
  n3 = Divide(x=w152, y=u16 2) -> (x/y=w147:dbl)
  n4 = Subtract(x=w145, y=w147) -> (x-y=w143:dbl)
  n5 = Add(x=w146, y=w147) -> (x+y=w144:dbl)
  n6 = Divide(x=w149, y=w141) -> (x/y=w118:dbl)
  "x vel" <- w118
  n7 = Unbundle By Name("Constants") -> ("Trigger_ticks"=w127:u32, "RS height- Pix"=w61:u16, "SCMOS-LineSpeed [10µs]"=w60:dbl, "Wobbel-total"=w34:dbl)  [unwired: 4 out]
  n8 = Increment(x=w144) -> (x+1=w138:dbl)
  n9 = Multiply(x=w143, y=w149) -> (x*y=w192:dbl)
  n10 = Multiply(x=w144, y=w149) -> (x*y=w191:dbl)
  n11 = Subtract "MovedPix"(x=w138, y=w143) -> (x-y=w142:dbl)
  n12 = Add(x=w191, y=w190) -> (x+y=w189:dbl)
  "~xgalvoend" <- w189
  n13 = Add(x=w192, y=w190) -> (x+y=w148:dbl)
  "xgalvostart" <- w148
  n14 = Multiply "CamTicks"(x=w142, y=w141) -> (x*y=w140:dbl)
  n15 = Divide(x=w155, y=w151) -> (x/y=w112:dbl)
  "WobSubShift" <- w112
  n16 = Round Toward +Infinity(x=w140) -> (ceil(x): smallest int >= x=w139:dbl)
  n17 = Subtract(x=w148, y=w189) -> (x-y=w188:dbl)
  "~x-move" <- w188
  n18 = To Unsigned Long Integer "Cam-Ticks"(number=w139) -> (unsigned 32bit integer=w83:u32)
  "CamTics" <- w83
  n19 = Multiply(x=w61, y=w60) -> (x*y=w58:dbl)
  n20 = call "MoveTime.vi"("maxaccel"=w196, "maxspeed"=w199, "dist"=w112) -> ("expected duration"=w198:dbl)
  "expected  Wduration" <- w198
  n21 = call "MoveTime.vi"("maxaccel"=w195, "maxspeed"=w199, "dist"=w188) -> ("expected duration"=w197:dbl)
  "expected xduration" <- w197
  n22 = Unbundle By Name("User") -> ("NoOfPhaseImages"=w68:u16)
  n23 = Multiply(x=w118, y=w83) -> (x*y=w119:dbl)
  "xGalvoMove" <- w119
  n24 = Max & Min(x=w198, y=w197) -> (max(x,y)=w63:dbl)  [unwired: 1 out]
  n25 = Unbundle By Name("Constants") -> ("extra-xgalvo"=w72:dbl)
  n26 = Max & Min(x=w54, y=w63) -> (max(x,y)=w62:dbl)  [unwired: 1 out]
  n27 = Multiply(x=w200, y=w151) -> (x*y=w217:u16)
  n28 = Divide(x=w62, y=u32 2) -> (x/y=w187:dbl)
  n29 = Divide(x=w72, y=w68) -> (x/y=w69:dbl)
  n30 = To Unsigned Long Integer(number=w187) -> (unsigned 32bit integer=w71:u32)
  "Half Turn_ticks" <- w71
  n31 = Multiply(x=w58, y=w193) -> (x*y=w59:dbl)
  n32 = Subtract(x=w119, y=w69) -> (x-y=w73:dbl)
  n33 = Compound Arithmetic op=ADD(w71, w71, w83) -> (w55:u32)
  "FrameClock" <- w55
  n34 = Unbundle By Name("Constants") -> ("zcommand"=w64:T3)
  n35 = formula code="a=(-x-2*v*t)/(t*(t-0));"("x"=w73, "v"=w118, "t"=w71) -> ("a"=w117:dbl)
  "galvo a" <- w117
  n36 = formula code="a=x/(t*(t-0));"("x"=w112, "t"=w71) -> ("a"=w113:dbl)
  "phase a" <- w113
  n37 = Divide(x=100000.0, y=w55) -> (x/y=w53:dbl)
  n38 = Bundle By Name(cluster=T2 {"Camera-Expos ms"=2499.6, "CameraImages"=70, "cam fps min."=9.518370454978108} ("Camera"), "Camera-Expos ms"=w59, "CameraImages"=w217, "cam fps min."=w53) -> (→"Camera":T2)
  n39 = Negate(x=w34) -> (-x=w33:dbl)
  n40 = Negate(x=w155) -> (-x=w57:dbl)
  n41 = Unbundle By Name("User") -> ("Digital-out"=w95:T10)
  n42 = call "SIAM-TMSI.vi"("Type"=enum8{"acc", "vel", "abs", "offset"}."abs", "Motor"=T7."x-Galvo") -> ("Resolution-Factor"=w179:i32, "command"=w180:T3)  [unwired: 6 in, 2 out]
  n43 = Subtract(x=w83, y=w82) -> (x-y=w128:u32)
  n44 = Unbundle By Name("User") -> ("Digital-out"=w132:T10)
  n45 = Multiply(x=w151, y=w210) -> (x*y=w203:i32)
  n46 = Add(x=u32 51, y=w35) -> (x+y=w31:u32)
  n47 = Subtract(x=w128, y=w127) -> (x-y=w87:u32)
  n48 = Divide(x=w33, y=w31) -> (x/y=w32:dbl)
  n49 = Decrement "z-step"(x=w203) -> ()  [unwired: 1 out]
  n50 = Boolean To (0,1)(Boolean=FALSE) -> (0, 1=w97:i16)
  n51 = Multiply(x=w71, y=w162) -> (x*y=w163:u32)
  n52 = call "SIAM-TMSI.vi"("Type"=enum8{"acc", "vel", "abs", "offset"}."acc", "Motor"=T7."x-Galvo") -> ("Resolution-Factor"=w121:i32, "command"=w103:T3)  [unwired: 6 in, 2 out]
  n53 = call "SIAM-TMSI.vi"("Type"=enum8{"acc", "vel", "abs", "offset"}."vel", "Motor"=T7."x-Galvo") -> ("Resolution-Factor"=w169:i32, "command"=w166:T3)  [unwired: 6 in, 2 out]
  n54 = call "SIAM-TMSI.vi"("Type"=enum8{"acc", "vel", "abs", "offset"}."acc", "Motor"=T7."Ch1") -> ("Resolution-Factor"=w114:i32, "command"=w102:T3)  [unwired: 6 in, 2 out]
  n55 = Boolean To (0,1)(Boolean=TRUE) -> (0, 1=w134:i16)
  n56 = To Unsigned Long Integer(number=w97) -> (unsigned 32bit integer=w96:u32)
  n57 = call "SIAM-TMSI.vi"("Type"=enum8{"acc", "vel", "abs", "offset"}."vel", "Motor"=T7."Ch1") -> ("Resolution-Factor"=w40:i32, "command"=w39:T3)  [unwired: 6 in, 2 out]
  n58 = call "SIAM-TMSI.vi"("Type"=enum8{"acc", "vel", "abs", "offset"}."vel", "Motor"=T7."Ch1") -> ("Resolution-Factor"=w47:i32, "command"=w46:T3)  [unwired: 6 in, 2 out]
  n59 = call "SIAM-TMSI.vi"("Type"=enum8{"acc", "vel", "abs", "offset"}."vel", "Motor"=T7."x-Galvo") -> ("Resolution-Factor"=w78:i32, "command"=w77:T3)  [unwired: 6 in, 2 out]
  n60 = call "SIAM-TMSI.vi"("Type"=enum8{"acc", "vel", "abs", "offset"}."abs", "Motor"=T7."Ch1") -> ("Resolution-Factor"=w174:i32, "command"=w175:T3)  [unwired: 6 in, 2 out]
  n61 = To Unsigned Long Integer(number=w134) -> (unsigned 32bit integer=w133:u32)
  n62 = Divide(x=w57, y=2) -> (x/y=w154:dbl)
  n63 = Multiply(x=w169, y=w118) -> (x*y=w170:dbl)
  n64 = Bundle By Name(cluster=w21, "Delay 10µs"=u32 50, "command"=w64, "P0"=w66, "comment"="z-shift") -> (w205:T8)
  n65 = Logical Shift(y=w95, x=u32 1) -> (x << y=w94:u32)
  n66 = Logical Shift(y=w95, x=w96) -> (x << y=w93:u32)
  n67 = Multiply(x=w179, y=w148) -> (x*y=w178:dbl)
  n68 = Multiply(x=w121, y=w117) -> (x*y=w109:dbl)
  n69 = Multiply(x=w114, y=w113) -> (x*y=w107:dbl)
  n70 = Multiply(x=w40, y=0) -> (x*y=w41:i32)
  n71 = Multiply(x=w47, y=w32) -> (x*y=w48:dbl)
  n72 = Logical Shift(y=w132, x=u32 1) -> (x << y=w131:u32)
  n73 = Multiply(x=w174, y=w154) -> (x*y=w173:dbl)
  n74 = Logical Shift(y=w132, x=w133) -> (x << y=w130:u32)
  n75 = Negate(x=w107) -> (-x=w108:dbl)
  n76 = Negate(x=w109) -> (-x=w110:dbl)
  n77 = Multiply(x=w78, y=0) -> (x*y=w79:i32)
  n78 = Bundle By Name(cluster=w21, "Delay 10µs"=w163, "command"=w166, "P2"=w170, "comment"="first line ramp") -> (w89:T8)
  n79 = Bundle By Name(cluster=w21, "Delay 10µs"=u32 0, "command"=w99, "P0"=w94, "P1"=w93, "comment"="laser off") -> (w85:T8)
  n80 = Bundle By Name(cluster=w21, "Delay 10µs"=u32 0, "command"=w185, "P0"=w183, "P1"=w151, "comment"="var2, raw counter") -> (w91:T8)
  n81 = Bundle By Name(cluster=w21, "Delay 10µs"=u32 0, "command"=w39, "P2"=w41) -> (w36:T8)
  n82 = Bundle By Name(cluster=w21, "Delay 10µs"=u32 0, "command"=w175, "P1"=w173, "comment"="shift start pos, sorry jump") -> (w150:T8)
  n83 = Bundle By Name(cluster=w21, "Delay 10µs"=w87, "command"=w103, "P3"=w109, "comment"="end linear, parabolic turn") -> (w120:T8)
  n84 = Bundle By Name(cluster=w21, "Delay 10µs"=u32 0, "command"=w180, "P1"=w178, "comment"="line startpos, jump") -> (w137:T8)
  n85 = Bundle By Name(cluster=w21, "Delay 10µs"=u32 0, "command"=w214, "P0"=w212, "P1"=w200, "comment"="var 3, z counter") -> (w206:T8)
  n86 = Bundle By Name(cluster=w21, "Delay 10µs"=u32 0, "command"=w46, "P2"=w48) -> (w44:T8)
  n87 = Bundle By Name(cluster=w21, "Delay 10µs"=u32 0, "command"=w161, "P0"=w156, "P1"=w160, "P2"=w157, "P5-ticket"=514, "comment"="raw loop") -> (w90:T8)
  n88 = Bundle By Name(cluster=w21, "command"=w102, "P3"=w107, "comment"="shift a") -> (w111:T8)
  n89 = Bundle By Name(cluster=w21, "Delay 10µs"=u32 0, "command"=w77, "P2"=w79) -> (w74:T8)
  n90 = Bundle By Name(cluster=w21, "Delay 10µs"=w71, "command"=w103, "P3"=w110, "comment"="decelerate line") -> (w106:T8)
  n91 = Bundle By Name(cluster=w21, "Delay 10µs"=w71, "command"=w103, "P3"=w101, "comment"="linear line") -> (w86:T8)
  n92 = Bundle By Name(cluster=w21, "command"=w102, "P3"=w108, "comment"="decerlaerate shift") -> (w105:T8)
  n93 = Bundle By Name(cluster=w21, "Delay 10µs"=w82, "command"=w136, "P0"=w131, "P1"=w130, "comment"="light on, linear here, loop point") -> (w126:T8)
  n94 = Bundle By Name(cluster=w21, "command"=w168, "P0"=w23, "P1"=w23, "comment"="cameras up") -> (w125:T8)
  n95 = Bundle By Name(cluster=w21, "command"=w102, "P3"=w101) -> (w100:T8)
  n96 = Bundle By Name(cluster=w125, "Delay 10µs"=w127, "P1"=0, "comment"="cameras down") -> (w124:T8)
  n97 = Multiply(x=w66, y=w200) -> (x*y=w220:i32)
  n98 = call "SIAM-TMSI.vi"("Type"=enum8{"acc", "vel", "abs", "offset"}."abs", "Motor"=T7."x-Galvo") -> ("Resolution-Factor"=w228:i32)  [unwired: 6 in, 3 out]
  n99 = Negate(x=w220) -> (-x=w65:i32)
  n100 = Multiply(x=w228, y=w218) -> (x*y=w229:dbl)
  n101 = Bundle By Name(cluster=w21, "Delay 10µs"=u32 50, "command"=w64, "P0"=w65, "comment"="go back z at end") -> (w219:T8)
  n102 = Bundle By Name(cluster=w21, "Delay 10µs"=w35, "command"=w211, "P0"=-19, "P1"=w209, "P2"=w207, "P5-ticket"=515, "comment"="z-loop") -> (w204:T8)
  n103 = Bundle By Name(cluster=w21, "Delay 10µs"=u32 1, "command"=w29, "P1"=w229, "comment"="stopp line, goto blanking") -> (w226:T8)
  n104 = Bundle By Name(cluster=w21, "Delay 10µs"=u32 1, "command"=w27, "P2"=w24, "P3"=w24, "comment"="stop phase") -> (w25:T8)
  n105 = Bundle By Name(cluster=w21, "Delay 10µs"=u32 10, "command"=w225, "P5-ticket"=368) -> (w26:T8)
  n106 = Build Array(w150, w36, w137, w89) -> (w202:T6)
  n107 = Build Array(w91, w126, w125, w124, w120, w111, w106, w105, w85, w86, w100, w90, w74, w44) -> (w104:T6)
  n108 = Build Array (concatenate)(w206, w202, w104, w205, w204, w219, w226, w25, w26) -> (w22:T6)
  "SIAMScript" <- w22
  n109 = Array Size(array=w22) -> (size(s)=→"size(s)":i32)
  n110 = case shown="True" "calulate values for debug" {
    tunnel: w22 -> [_ w233]
    frame False {
    }
    frame True {
      # "old format without comment"
      n111 = for {
        tunnel: w233 -> [w238] mode=indexing
        tunnel: [w239] -> w232 mode=indexing
        n112 = Unbundle(w238) -> ("Delay 10µs"=w247:u32, "command"=w246:T3, "P0"=w245:i32, "P1"=w244:i32, "P2"=w243:i32, "P3"=w242:i32, "P4"=w241:i32, "P5-ticket"=w240:i32)  [unwired: 1 out]
        n113 = Bundle("Delay 10µs"=w247, "command"=w246, "P0"=w245, "P1"=w244, "P2"=w243, "P3"=w242, "P4"=w241, "P5-ticket"=w240) -> (w239:T11)  [unwired: 1 in]
      }
      n114 = call "SIAM_to_ScanControl.vi"("Script"=w232) -> ("ScanSteuerung"=w237:T14)  [unwired: 8 in, 2 out]
      n115 = call "ScanSteuerung_to_Datapoints.vi"("ScanSteuerung"=w237, "Aktiv"="Aktiv", "Neues Zeitraster"=1.0) -> ("Waveform Graph"=→"Waveform Graph":dbl[][])  [unwired: 1 in, 1 out]
    }
  }
  "error out" <- "error in (no error)"
